vi "Auto备份.vi"() -> ()   [LabVIEW 2019]
uses:
  Global_Variable/A180648.vi
  Global_Variable/Global.vi
  Libraries/S7/S7.lvlib
  <userlib>/_MGI/1D Array/MGI Running Average/MGI Running Average(DBL).vi
  <userlib>/_MGI/1D Array/MGI Running Average/MGI Running Average(SGL).vi
  <userlib>/_MGI/1D Array/MGI Running Average/MGI Running Average(DBL[]).vi
panel:
  out "试验项_Event":refnum<user-event>
  out "NVH":bool=TRUE
  out "T1+T2":dbl
  out "T2":dbl
  out "T1":dbl
  out "吸收电流":sgl
  out "输出扭矩(大)":sgl
  out "输入扭矩":sgl
  out "力特性逆向去程":bool
  out "力特性正向去程":bool
  out "力特性逆向回程":bool
  out "力特性正向回程":bool
  out "逆向空载正向初始化":bool
  out "锁紧/开启初始化":bool
  out "功能正向初始化":bool
  out "功能逆向初始化":bool
  out "空载逆向初始化":bool
  out "空载正向初始化":bool
  out "布尔":bool=TRUE
  out "当前车速":i32
  out "试验项目":T1(tab)
  out "手柄锁紧力试验":cluster{dbl[], dbl[]}[](graph)
  out "手柄开启力试验":cluster{dbl[], dbl[]}[](graph)
  out "管柱推拉力试验":cluster{dbl[], dbl[]}[](graph)
  out "管柱保持力试验":cluster{dbl[], dbl[]}[](graph)
  out "锁紧/开启":cluster{dbl[], dbl[]}[](graph)
  out "逆向空载试验":cluster{dbl[], dbl[]}[](graph)
  out "振动2NHV-FFT":cluster{"f0":dbl, "df":dbl, "magnitude":dbl[]}[](graph)
  out "振动1NVH-FFT":cluster{"f0":dbl, "df":dbl, "magnitude":dbl[]}[](graph)
  in  "判定结果":bool[][](array[boolean])=[[TRUE]]
  in  "STEP":string
  # "车速1"
  # "车速2"
  # "车速3"
  # "车速4"
  # "车速5"
  # "车速6"
  # "车速1"
  # "车速2"
  # "车速3"
  # "车速4"
  # "车速5"
  # "车速6"
  # "."
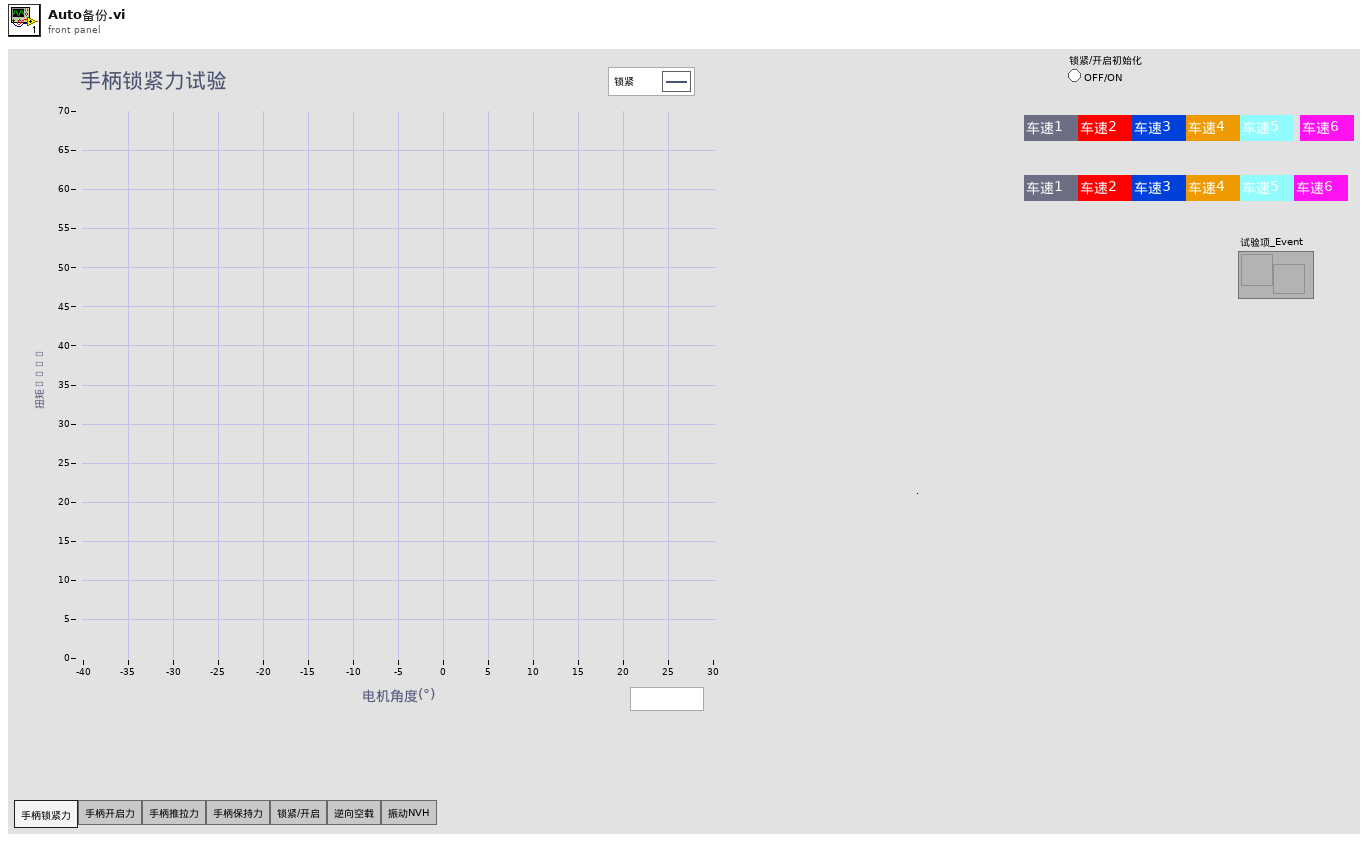
[diagram p1: front panel]
types:
  T1 = enum32{"手柄锁紧力", "手柄开启力", "手柄推拉力", "手柄保持力", "锁紧/开启", "逆向空载", "振动NVH"}
  T2 = enum32{"Invalid", "Standard", "Closed", "Hidden", "Minimized", "Maximized"}
  T3 = enum32{"手柄锁紧力", "手柄开启力", "手柄推拉力", "手柄保持力", "锁紧/开启", "逆向空载", "振动NVH", "完成"}
  T4 = cluster{"输入轴扭矩":dbl, "输出轴扭矩小量程":dbl, "输出轴扭矩大量程":dbl}
  T5 = cluster{"锁紧判断范围":cluster{"单位":string, "下限":dbl, "上限":dbl}}
  T6 = cluster{"开启判断范围":cluster{"单位":string, "下限":dbl, "上限":dbl}}
  T7 = cluster{"推拉力判断范围 ":cluster{"单位":string, "下限":dbl, "上限":dbl}}
  T8 = cluster{"保持力判断范围 ":cluster{"单位":string, "下限":dbl, "上限":dbl}, "保持力监控位移":cluster{"单位":string, "下限":dbl, "上限":dbl}}
  T9 = cluster{"输入旋转位移":sgl, "输入移载位移":sgl, "工装移载位移":sgl, "输入编码位移":sgl, "输入扭矩":sgl, "输出扭矩(小)":sgl, "输出扭矩(大)":sgl, "吸收电流":sgl}
  T10 = typedef "svc_Spectrum Info.ctl" = cluster{"channel name":string, "description":string, "x-axis units":T11, "spectral info":cluster{"spectrum type":T12, "linear/dB":enum16{"linear", "dB"}, "window":u16, "window size":i32, "FFT size":i32}, "engineering units":T13, "custom label":string, "dB reference [EU]":dbl, "peak units":enum16{"rms", "peak", "peak-peak"}, "weighting filter":T14, "spectral density?":bool, "unit label":string, "spectrum skewed?":bool, "complimentary spectrum units":T15}
  T11 = typedef "svc_X-Axis Units.ctl" = u16
  T12 = typedef "svc_Spectrum Type.ctl" = enum16{"FFT Spectrum [complex]", "Amplitude [Magnitude]", "Power [Magnitude^2]", "Cross Spectrum [complex]", "Frequency Response [Complex]"}
  T13 = typedef "svc_Engineering Units Text Ring.ctl" = u16
  T14 = typedef "svc_Weighting Filter Text Ring.ctl" = u16
  T15 = typedef "svc_Complimentary Spectrum Units.ctl" = enum16{"none", "radians", "degrees", "cycles", "imaginary"}
  T16 = cluster{"启用助力":dbl, "试验速度":dbl, "试验角度":dbl, "保护扭矩":dbl}
  T17 = typedef "lveventtype.ctl" = enum32{"Null", "Timeout", "Annotation Menu Selection", "Annotation Menu Selection?", "App Instance Close", "App Instance Close?", "Autoscale Range Change", "Bookmark Info Change", "Cell Edit", "Cell Edit?", "Cursor Grab", "Cursor Grab?", "Cursor Menu Selection", "Cursor Menu Selection?", "Cursor Move", "Cursor Release", "Data Change", "Direction Change", "Display State Change", "Drag Ended", "Drag Enter", "Drag Leave", "Drag Over", "Drag Source Update", "Drag Starting", "Drag Starting?", "Drop", "Exec State Change", "Key Down", "Key Down?", "Key Repeat", "Key Repeat?", "Key Up", "Listbox Double Click", "Menu Activation?", "Menu Selection (App)", "Menu Selection? (App)", "Menu Selection (User)", "Mouse Down", "Mouse Down?", "Mouse Enter", "Mouse Leave", "Mouse Move", "Mouse Up", "Mouse Wheel", "NI Security User Change (App)", "Pane Size", "Panel Close", "Panel Close?", "Panel Resize", "Plot Attribute Change", "Scale Range Change", "Shortcut Menu Activation?", "Shortcut Menu Selection (App)", "Shortcut Menu Selection? (App)", "Shortcut Menu Selection (User)", "Tree Double Click", "Tree Drag", "Tree Drag?", "Tree Drop", "Tree Drop?", "Tree Item Close", "Tree Item Close?", "Tree Item Open", "Tree Item Open?", "User Event", "Value Change"}
  T18 = typedef "LVPoint32TypeDef.ctl" = cluster{"Horizontal":i32, "Vertical":i32}
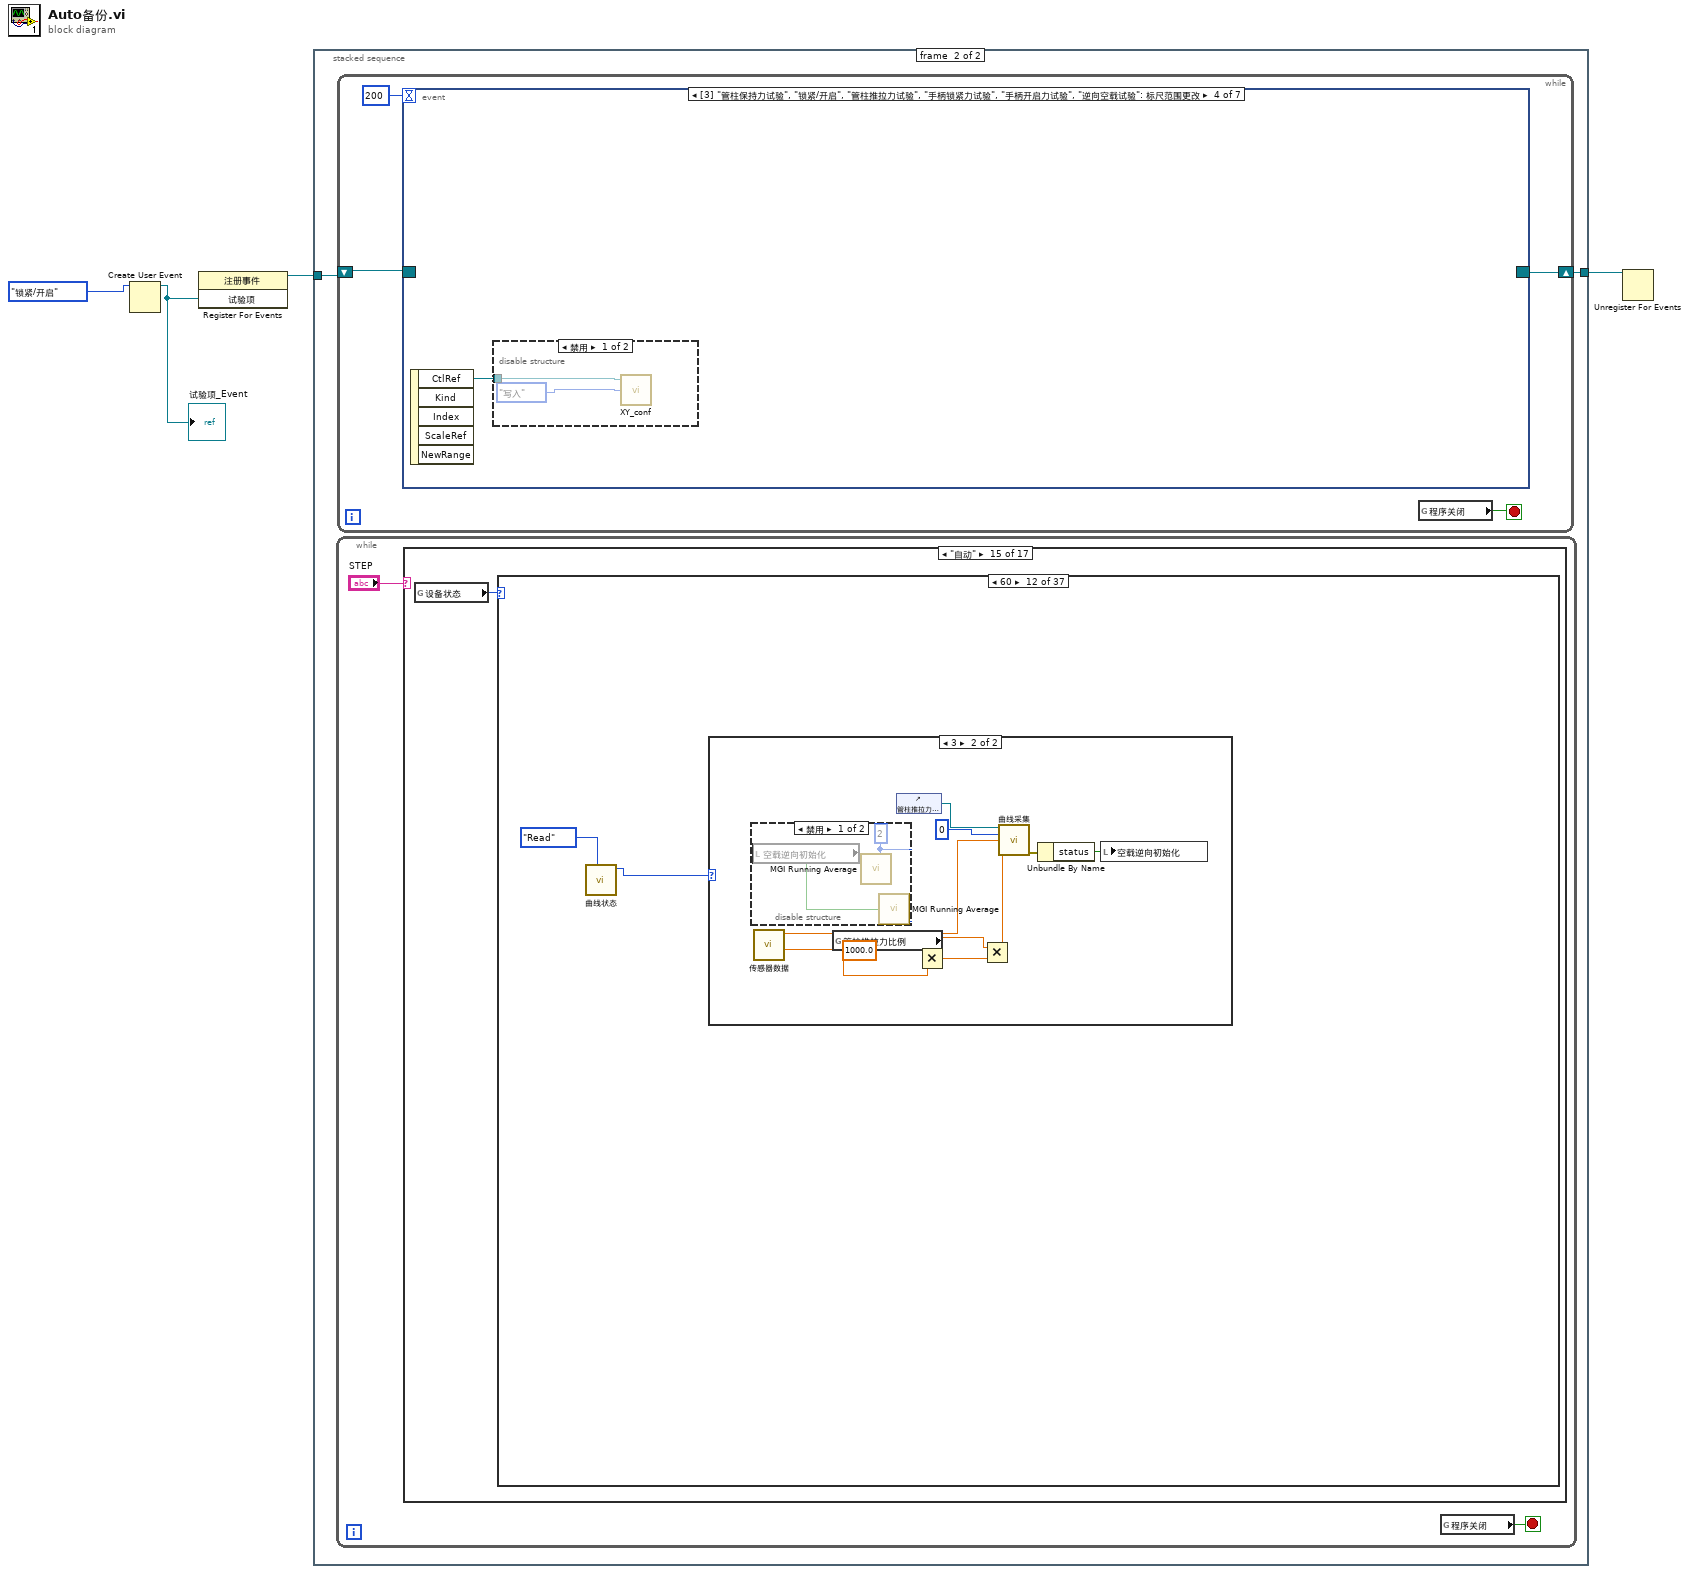
[diagram p0: block diagram]
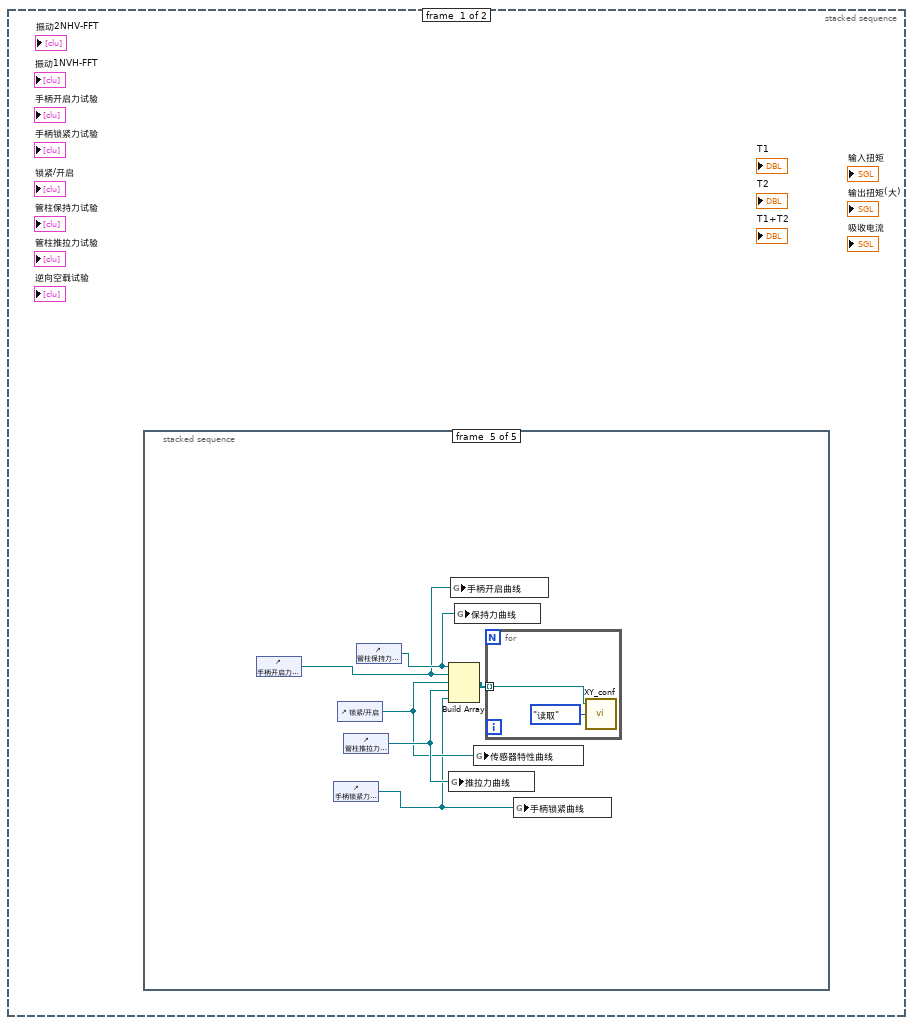
[diagram p2: hidden frame]
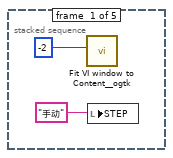
[diagram p3: hidden frame]
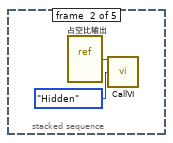
[diagram p4: hidden frame]
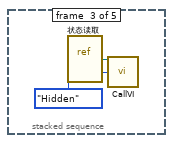
[diagram p5: hidden frame]
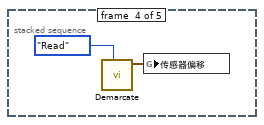
[diagram p6: hidden frame]
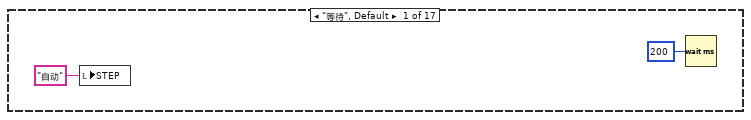
[diagram p7: hidden frame]
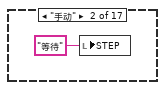
[diagram p8: hidden frame]
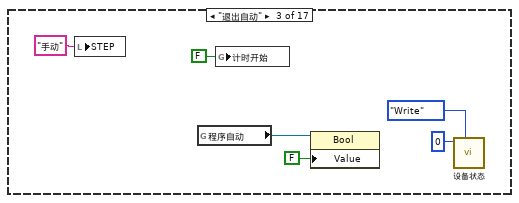
[diagram p9: hidden frame]
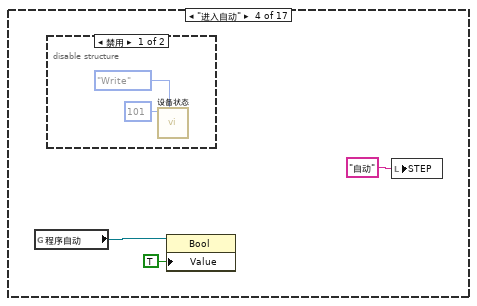
[diagram p10: hidden frame]
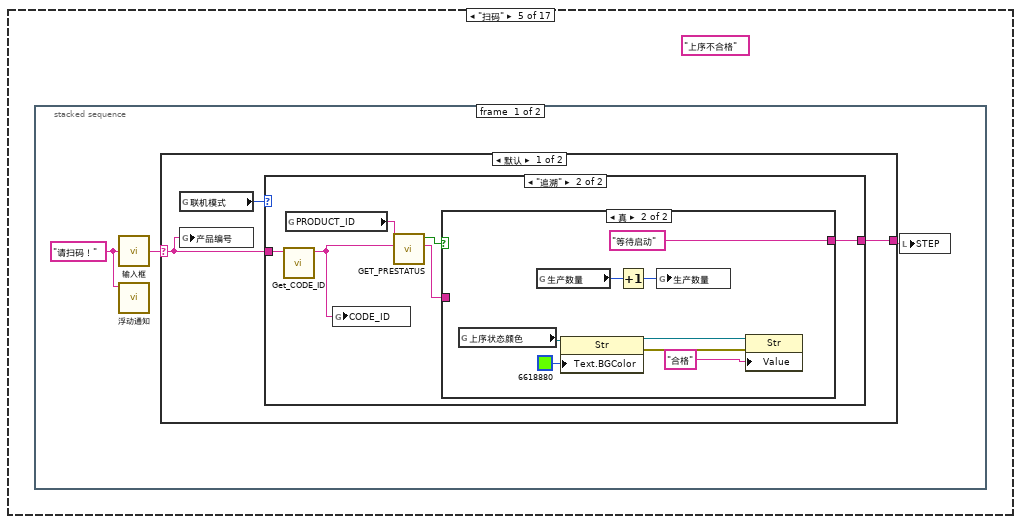
[diagram p12: hidden frame]
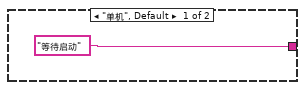
[diagram p13: hidden frame]
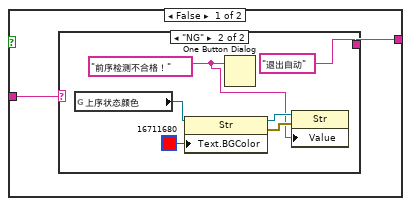
[diagram p14: hidden frame]
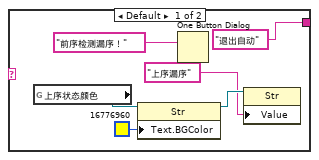
[diagram p15: hidden frame]
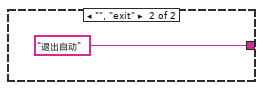
[diagram p16: hidden frame]
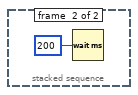
[diagram p17: hidden frame]
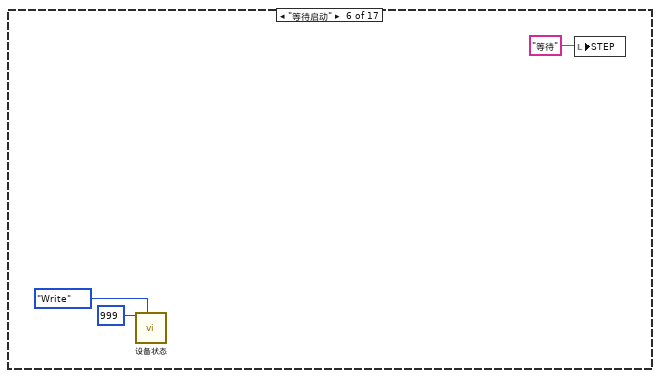
[diagram p18: hidden frame]
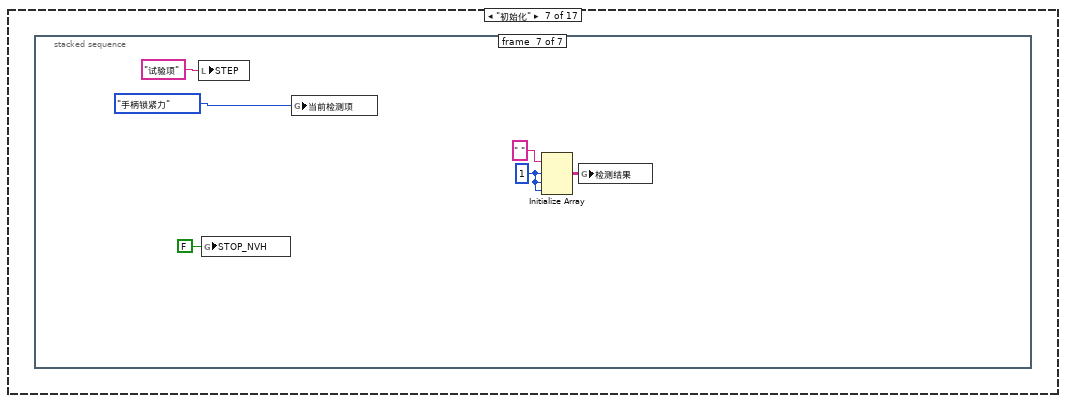
[diagram p19: hidden frame]
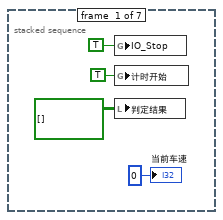
[diagram p20: hidden frame]
diagram:
  n1 = Create User Event(user event datatype=T1."锁紧/开启" ("试验项")) -> (user event=w1:refnum<user-event>)  [unwired: 1 in, 1 out]
  "试验项_Event" <- w1
  n2 = register-events(w1) -> (reference out=w2:refnum<event-registration>)  [unwired: 2 in, 1 out]
  n3 = stacked-sequence {
    tunnel: [_ w22] -> w4
    tunnel: w2 -> [_ w21]
    frame #0 {
      n4 = stacked-sequence {
        frame #0 {
          n5 = call <userlib>:"Fit VI window to Content__ogtk.vi"("border spacing (2 px)"=-2) -> ()  [unwired: 5 in, 2 out]
          n6 = local write "STEP"("手动" ("STEP")) -> ()
        }
        frame #1 {
          n7 = vi-ref "占空比输出.vi"() -> (w8:refnum<vi>)
          n8 = call "CallVI.vi"("VI引用"=w8, "状态"=T2."Hidden") -> ()  [unwired: 12 in, 2 out]
        }
        frame #2 {
          n9 = vi-ref "状态读取.vi"() -> (w10:refnum<vi>)
          n10 = call "CallVI.vi"("VI引用"=w10, "状态"=T2."Hidden") -> ()  [unwired: 12 in, 2 out]
        }
        frame #3 {
          n11 = call "Demarcate.vi"("Mode"=enum16{"Read", "Write"}."Read") -> ("Sensor OUT"=w12:T4)  [unwired: 9 in, 1 out]
          n12 = global write "传感器偏移.vi" "传感器偏移"(w12) -> ()
        }
        frame #4 {
          n13 = control-ref of="手柄开启力试验"() -> (w14:refnum<vi>)
          n14 = control-ref of="手柄锁紧力试验"() -> (w13:refnum<vi>)
          n15 = control-ref of="锁紧/开启"() -> (w15:refnum<vi>)
          n16 = control-ref of="管柱推拉力试验"() -> (w18:refnum<vi>)
          n17 = control-ref of="管柱保持力试验"() -> (w16:refnum<vi>)
          n18 = Build Array(w16, w14, w15, w18, w13) -> (w17:refnum<vi>[])
          n19 = global write "A180648.vi" "推拉力曲线"(w18) -> ()
          n20 = global write "A180648.vi" "手柄开启曲线"(w14) -> ()
          n21 = global write "A180648.vi" "保持力曲线"(w16) -> ()
          n22 = global write "A180648.vi" "传感器特性曲线"(w15) -> ()
          n23 = for {
            tunnel: w17 -> [w19] mode=indexing
            n24 = call "XY_conf.vi"("方式"=enum16{"写入", "读取"}."读取", "XY图引用"=w19) -> ()  [unwired: 3 in, 1 out]
          }
          n25 = global write "A180648.vi" "手柄锁紧曲线"(w13) -> ()
        }
      }
    }
    frame #1 {
      n26 = while {
        stop <- w24 stop-if-true
        n27 = case shown="\"自动\"" "STEP" {
          frame "等待", Default {
            n28 = local write "STEP"("自动" ("STEP")) -> ()
            n29 = Wait (ms)(milliseconds to wait=u32 200 ("等待时间（毫秒）")) -> ()  [unwired: 1 out]
          }
          frame "手动" {
            n30 = local write "STEP"("等待" ("STEP")) -> ()
          }
          frame "退出自动" {
            n31 = local write "STEP"("手动" ("STEP")) -> ()
            n32 = global read "Global.vi" "程序自动"() -> (w29:refnum<vi>)
            n33 = global write "Global.vi" "计时开始"(FALSE ("计时开始")) -> ()
            n34 = property class="Bool"(reference=w29, "Value"=FALSE) -> ()  [unwired: 1 in, 2 out]
            n35 = call "设备状态.vi"("枚举"=enum16{"Read", "Write"}."Write", "Status_Write"=i16 0) -> ()  [unwired: 9 in, 1 out]
          }
          frame "进入自动" {
            n36 = global read "Global.vi" "程序自动"() -> (w35:refnum<vi>)
            n37 = disable-structure shown="禁用" {
              frame Disabled {
                n38 = call "设备状态.vi"("枚举"=enum16{"Read", "Write"}."Write", "Status_Write"=i16 101) -> ()  [unwired: 9 in, 1 out]
              }
              frame Enabled {
              }
            }
            n39 = property class="Bool"(reference=w35, "Value"=TRUE) -> ()  [unwired: 1 in, 2 out]
            n40 = local write "STEP"("自动" ("STEP")) -> ()
          }
          frame "扫码" {
            (unwired) "上序不合格" ("上序状态")
            n41 = stacked-sequence {
              frame #0 {
                w40 = "请扫码！" ("提示信息")
                n42 = call "输入框.vi"("提示信息"=w40) -> ("条形码输出"=w41:string)
                n43 = call "浮动通知.vi"("通知内容"=w40) -> ()  [unwired: 11 in]
                n44 = case shown="默认" w41 {
                  selector: w41 -> [w43 _]
                  tunnel: [w44 "退出自动" ("State(s) in Front (\"\")")] -> w39
                  frame Default {
                    n45 = global read "Global.vi" "联机模式"() -> (w42:enum16{"单机", "追溯"})
                    n46 = global write "Global.vi" "产品编号"(w43) -> ()
                    n47 = case shown="\"追溯\"" w42 {
                      tunnel: ["等待启动" ("State(s) in Front (\"\")") w51] -> w44
                      tunnel: w43 -> [_ w48]
                      frame "单机", Default {
                      }
                      frame "追溯" {
                        n48 = call "Get_CODE_ID.vi"("CODE_MAIN"=w48) -> ("CODE_ID"=w47:string)  [unwired: 10 in]
                        n49 = global read "追溯Global.vi" "PRODUCT_ID"() -> (w50:string)
                        n50 = global write "追溯Global.vi" "CODE_ID"(w47) -> ()
                        n51 = call "GET_PRESTATUS.vi"("CODE_ID"=w47, "PRODUCT_ID"=w50) -> ("字符串"=w46:string, "OK?"=w49:bool)  [unwired: 8 in]
                        n52 = case shown="真" w49 {
                          tunnel: [w53 "等待启动" ("State(s) in Front (\"\")")] -> w51
                          tunnel: w46 -> [w52 _]
                          frame False {
                            n53 = case shown="\"NG\"" w52 {
                              tunnel: ["退出自动" ("State(s) in Front (\"\")") "退出自动" ("State(s) in Front (\"\")")] -> w53
                              frame Default {
                                n54 = global read "Global.vi" "上序状态颜色"() -> (w59:refnum<vi>)
                                n55 = property class="Str"(reference=w59, "Text.BGColor"=u32 16776960 ("文本.文本颜色:背景色")) -> (reference out=w55:refnum<vi>)  [unwired: 1 in, 1 out]
                                n56 = One Button Dialog(message="前序检测漏序！" ("消息")) -> ()  [unwired: 1 in, 1 out]
                                n57 = property class="Str"(reference=w55, "Value"="上序漏序" ("上序状态")) -> ()  [unwired: 1 in, 2 out]
                              }
                              frame "NG" {
                                w60 = "前序检测不合格！" ("消息")
                                n58 = global read "Global.vi" "上序状态颜色"() -> (w64:refnum<vi>)
                                n59 = property class="Str"(reference=w64, "Text.BGColor"=u32 16711680 ("文本.文本颜色:背景色")) -> (reference out=w62:refnum<vi>, error out=w61:errorcluster)  [unwired: 1 in]
                                n60 = One Button Dialog(message=w60) -> ()  [unwired: 1 in, 1 out]
                                n61 = property class="Str"(reference=w62, error in=w61, "Value"=w60) -> ()  [unwired: 2 out]
                              }
                            }
                          }
                          frame True {
                            n62 = global read "Global.vi" "上序状态颜色"() -> (w70:refnum<vi>)
                            n63 = global read "Global.vi" "生产数量"() -> (w71:i32)
                            n64 = property class="Str"(reference=w70, "Text.BGColor"=u32 6618880 ("文本.文本颜色:背景色")) -> (reference out=w68:refnum<vi>, error out=w67:errorcluster)  [unwired: 1 in]
                            n65 = Increment(x=w71) -> (x+1=w72:i32)
                            n66 = global write "Global.vi" "生产数量"(w72) -> ()
                            n67 = property class="Str"(reference=w68, error in=w67, "Value"="合格" ("上序状态")) -> ()  [unwired: 2 out]
                          }
                        }
                      }
                    }
                  }
                  frame "", "exit" {
                  }
                }
                n68 = local write "STEP"(w39) -> ()
              }
              frame #1 {
                n69 = Wait (ms)(milliseconds to wait=u32 200 ("等待时间（毫秒）")) -> ()  [unwired: 1 out]
              }
            }
          }
          frame "等待启动" {
            n70 = call "设备状态.vi"("枚举"=enum16{"Read", "Write"}."Write", "Status_Write"=i16 999 ("设备状态")) -> ()  [unwired: 9 in, 1 out]
            n71 = local write "STEP"("等待" ("STEP")) -> ()
          }
          frame "初始化" {
            n72 = stacked-sequence {
              frame #0 {
                n73 = global write "Global.vi" "IO_Stop"(TRUE ("IO_Stop")) -> ()
                n74 = global write "Global.vi" "计时开始"(TRUE ("计时开始")) -> ()
                n75 = local write "判定结果"(bool[][] [] ("判定结果")) -> ()
                "当前车速" <- 0 ("当前车速")
              }
              frame #1 {
                w86 = TRUE
                n76 = global read "Global.vi" "试验项目"() -> (w85:bool[])
                n77 = Index Array(array=w85, index=4 ("索引")) -> (element=w83:bool)
                n78 = case shown="假" w83 {
                  frame False {
                    n79 = local write "锁紧/开启初始化"(FALSE ("锁紧/开启初始化")) -> ()
                  }
                  frame True {
                    "锁紧/开启初始化" <- TRUE ("锁紧/开启初始化")
                  }
                }
                "逆向空载正向初始化" <- w86
                "空载正向初始化" <- w86
                "空载逆向初始化" <- w86
                "功能正向初始化" <- w86
                "功能逆向初始化" <- w86
                "力特性逆向去程" <- w86
                "力特性正向去程" <- w86
                "力特性逆向回程" <- w86
                "力特性正向回程" <- w86
              }
              frame #2 {
                n80 = for {
                  N: 24 -> [_]
                  tunnel: [cluster{dbl[], dbl[]} {[], []}] -> w90 mode=indexing
                  tunnel: [cluster{"f0":dbl, "df":dbl, "magnitude":dbl[]} {"f0"=0.0, "df"=0.0, "magnitude"=[]} ("power spectrum [dB EU]")] -> w89 mode=indexing
                }
                n81 = local write "管柱推拉力试验"(w90) -> ()
                n82 = local write "管柱保持力试验"(w90) -> ()
                n83 = local write "手柄锁紧力试验"(w90) -> ()
                n84 = local write "手柄开启力试验"(w90) -> ()
                n85 = local write "逆向空载试验"(w90) -> ()
                n86 = local write "锁紧/开启"(w90) -> ()
                n87 = local write "振动2NHV-FFT"(w89) -> ()
                n88 = local write "振动1NVH-FFT"(w89) -> ()
              }
              frame #3 {
                n89 = global read "Global.vi" "Result"() -> (w96:refnum<vi>)
                n90 = property class="Tbl"(reference=w96, "Value"=string[][] []) -> (reference out=w97:refnum<vi>, error out=w98:errorcluster)  [unwired: 1 in]
                n91 = property class="Tbl"(reference=w97, error in=w98, "Row Headers[]"=string[] [] ("列首字符串[]")) -> ()  [unwired: 2 out]
              }
              frame #4 {
                n92 = global read "A180648.vi" "LED-手柄锁紧力"() -> (w100:refnum<vi>)
                n93 = global read "A180648.vi" "LED-手柄开启力"() -> (w101:refnum<vi>)
                n94 = global read "A180648.vi" "LED-推拉力"() -> (w103:refnum<vi>)
                n95 = global read "A180648.vi" "LED-保持力"() -> (w99:refnum<vi>)
                n96 = Build Array(w100, w101, w103, w99) -> (w102:refnum<vi>[])
                n97 = for {
                  tunnel: w102 -> [w104] mode=indexing
                  n98 = property class="Bool"(reference=w104, "Colors [4]"=cluster{u32, u32}[] [{12369084, 12369084}] ("颜色[4]")) -> ()  [unwired: 1 in, 2 out]
                }
              }
              frame #5 {
                n99 = global read "Global.vi" "启用CAN"() -> (w106:bool)
                n100 = case shown="真" w106 {
                  frame False {
                  }
                  frame True {
                    n101 = call "循环发送CAN.vi"() -> ()  [unwired: 11 in, 1 out]
                  }
                }
              }
              frame #6 {
                w109 = 1 ("维数大小")
                n102 = local write "STEP"("试验项" ("STEP")) -> ()
                n103 = global write "Global.vi" "STOP_NVH"(FALSE ("STOP_NVH")) -> ()
                n104 = global write "A180648.vi" "当前检测项"(T3."手柄锁紧力" ("值(信号)")) -> ()
                n105 = Initialize Array(" " ("字符串"), w109, w109, w109) -> (w111:string[][][])
                n106 = global write "A180648.vi" "检测结果"(w111) -> ()
              }
            }
          }
          frame "试验项" {
            n107 = global read "A180648.vi" "当前检测项"() -> (w113:T3)
            n108 = case shown="\"完成\"" w113 {
              selector: w113 -> [w115 _]
              tunnel: [w118 "报表" ("STEP")] -> w114
              frame "手柄锁紧力", Default {
                n109 = global read "Global.vi" "试验项目"() -> (w116:bool[])
                n110 = Index Array(array=w116, index=w115) -> (element=w117:bool)
                n111 = case shown="真" w117 {
                  tunnel: ["试验项" ("字符串") w125] -> w118
                  tunnel: w115 -> [_ w126]
                  frame False {
                    n112 = global read "A180648.vi" "当前检测项"() -> (w123:T3)
                    n113 = Increment(x=w123) -> (x+1=w122:T3)
                    n114 = global write "A180648.vi" "当前检测项"(w122) -> ()
                    n115 = local read "判定结果"() -> (w119:bool[][])
                    n116 = Build Array (concatenate)(w119, bool[] [FALSE] ("判定结果")) -> (w120:bool[][])
                    n117 = local write "判定结果"(w120) -> ()
                  }
                  frame True {
                    n118 = case shown="\"手柄推拉力\"" w126 {
                      tunnel: ["手柄锁紧力" ("STEP") "手柄开启力" ("STEP") "手柄推拉力" ("STEP") "手柄保持力" ("STEP") "套输入轴花键" ("STEP") w153 "退输入轴花键" ("STEP")] -> w125
                      frame "手柄锁紧力", Default {
                        n119 = call "浮动通知.vi"("通知内容"="手柄锁紧力试验") -> ()  [unwired: 11 in]
                        n120 = property on="试验项目" class="TabCtl (严格)"("Val(Sgnl)"=T1."手柄锁紧力" ("值(信号)")) -> ()  [unwired: 2 in, 2 out]
                      }
                      frame "手柄开启力" {
                        n121 = call "浮动通知.vi"("通知内容"="手柄开启力试验") -> ()  [unwired: 11 in]
                        n122 = property on="试验项目" class="TabCtl (严格)"("Val(Sgnl)"=T1."手柄开启力" ("值(信号)")) -> ()  [unwired: 2 in, 2 out]
                      }
                      frame "手柄推拉力" {
                        n123 = call "浮动通知.vi"("通知内容"="管柱推拉力试验") -> ()  [unwired: 11 in]
                        n124 = property on="试验项目" class="TabCtl (严格)"("Val(Sgnl)"=T1."手柄推拉力" ("值(信号)")) -> ()  [unwired: 2 in, 2 out]
                      }
                      frame "手柄保持力" {
                        n125 = call "浮动通知.vi"("通知内容"="管柱保持力试验") -> ()  [unwired: 11 in]
                        n126 = property on="试验项目" class="TabCtl (严格)"("Val(Sgnl)"=T1."手柄保持力" ("值(信号)")) -> ()  [unwired: 2 in, 2 out]
                      }
                      frame "完成" {
                        n127 = for {
                          tunnel: sgl[] [1.0, 15.0] ("力特性参数") -> [w142] mode=indexing
                          i -> [w145]
                          w150 = u16 2 items=["byte", "word", "Dword"] ("数据类型")
                          w152 = u8 132 items=["I/O (P)"=128, "Input (I)"=129, "Output (Q)"=130, "Bit Memory (M)"=131, "Data (DB)"=132, "Instance Data (DI)"=133, "Local Data (L)"=134, "Predecessor Local Data (VL)"=135] ("寄存器类型")
                          n128 = Type Cast(type=u32 0 ("写入地址"), x=w142) -> (*(type *) &x=w148:u32)
                          n129 = Multiply(x=w145, y=4) -> (x*y=w146:i32)
                          n130 = Add(x=u32 152 ("写入地址"), y=w146) -> (x+y=w143:u32)
                          n131 = call "Write_Data.vi"("DB #"=u16 7, "寄存器类型"=w152, "写入数据"=w148, "数据类型"=w150, "写入地址"=w143) -> ()  [unwired: 4 in, 3 out]
                        }
                        n132 = call "浮动通知.vi"("通知内容"="传感器特性试验") -> ()  [unwired: 11 in]
                      }
                      frame "振动NVH" {
                        n133 = call "浮动通知.vi"("通知内容"="振动NVH试验") -> ()  [unwired: 11 in]
                        n134 = local read "NVH"() -> (w156:bool)
                        n135 = Select(t="判定" ("STEP"), s=w156, f="退输入轴花键" ("STEP")) -> (s? t:f=w153:string)
                      }
                      frame "逆向空载" {
                        n136 = call "浮动通知.vi"("通知内容"="逆向空载试验") -> ()  [unwired: 11 in]
                      }
                    }
                  }
                }
              }
              frame "完成" {
                n137 = call "浮动通知.vi"("通知内容"="试验完成") -> ()  [unwired: 11 in]
                n138 = call "设备状态.vi"("枚举"=enum16{"Read", "Write"}."Write", "Status_Write"=i16 100 ("设备状态")) -> ()  [unwired: 9 in, 1 out]
              }
            }
            n139 = local write "STEP"(w114) -> ()
          }
          frame "判定" {
            n140 = stacked-sequence {
              frame #0 {
                n141 = global read "A180648.vi" "当前检测项"() -> (w164:T3)
                n142 = case shown="\"手柄开启力\"" w164 {
                  frame "完成", Default {
                  }
                  frame "手柄锁紧力" {
                    n143 = global read "判定参数.vi" "锁紧判定参数"() -> (w176:T5)
                    n144 = local read "手柄锁紧力试验"() -> (w177:cluster{dbl[], dbl[]}[])
                    n145 = global read "A180648.vi" "LED-手柄锁紧力"() -> (w171:refnum<vi>)
                    n146 = global read "Global.vi" "Result"() -> (w175:refnum<vi>)
                    n147 = call "锁紧试验判定.vi"("Result"=w175, "判定参数"=w176, "XY曲线"=w177) -> ("判定项长度"=w166:i32, "OK？"=w165:bool)  [unwired: 7 in]
                    n148 = Select(t=cluster{u32, u32}[] [{6618880, 6618880}, {6618880, 6618880}, {6618880, 6618880}, {6618880, 6618880}] ("颜色[4]"), s=w165, f=cluster{u32, u32}[] [{16711680, 16711680}, {16711680, 16711680}, {16711680, 16711680}, {16711680, 16711680}] ("颜色[4]")) -> (s? t:f=w172:cluster{u32, u32}[])
                    n149 = property class="Bool"(reference=w171, "Colors [4]"=w172) -> ()  [unwired: 1 in, 2 out]
                    n150 = local read "判定结果"() -> (w167:bool[][])
                    n151 = Build Array(TRUE, w165) -> (w170:bool[])
                    n152 = global write "判定参数.vi" "锁紧判定长度"(w166) -> ()
                    n153 = Build Array (concatenate)(w167, w170) -> (w168:bool[][])
                    n154 = case shown="假" w165 {
                      frame False {
                        n155 = call "合格状态.vi"("枚举"=enum16{"Read", "Write"}."Write", "起始地址"=u32 180, "Status_Write"=i16 2) -> ()  [unwired: 8 in, 1 out]
                      }
                      frame True {
                        n156 = call "合格状态.vi"("枚举"=enum16{"Read", "Write"}."Write", "起始地址"=u32 180, "Status_Write"=i16 1) -> ()  [unwired: 8 in, 1 out]
                      }
                    }
                    n157 = local write "判定结果"(w168) -> ()
                  }
                  frame "手柄开启力" {
                    n158 = global read "A180648.vi" "LED-手柄开启力"() -> (w191:refnum<vi>)
                    n159 = global read "判定参数.vi" "开启判定参数"() -> (w196:T6)
                    n160 = local read "手柄开启力试验"() -> (w197:cluster{dbl[], dbl[]}[])
                    n161 = global read "Global.vi" "Result"() -> (w195:refnum<vi>)
                    n162 = call "开启试验判定.vi"("Result"=w195, "判定参数"=w196, "XY曲线"=w197) -> ("判定项长度"=w186:i32, "OK？"=w184:bool)  [unwired: 7 in]
                    n163 = Select(t=cluster{u32, u32}[] [{6618880, 6618880}, {6618880, 6618880}, {6618880, 6618880}, {6618880, 6618880}] ("颜色[4]"), s=w184, f=cluster{u32, u32}[] [{16711680, 16711680}, {16711680, 16711680}, {16711680, 16711680}, {16711680, 16711680}] ("颜色[4]")) -> (s? t:f=w192:cluster{u32, u32}[])
                    n164 = property class="Bool"(reference=w191, "Colors [4]"=w192) -> ()  [unwired: 1 in, 2 out]
                    n165 = local read "判定结果"() -> (w187:bool[][])
                    n166 = global write "判定参数.vi" "开启判定长度"(w186) -> ()
                    n167 = Build Array(TRUE, w184) -> (w190:bool[])
                    n168 = Build Array (concatenate)(w187, w190) -> (w188:bool[][])
                    n169 = case shown="假" w184 {
                      frame False {
                        n170 = call "合格状态.vi"("枚举"=enum16{"Read", "Write"}."Write", "起始地址"=u32 76, "Status_Write"=i16 2) -> ()  [unwired: 8 in, 1 out]
                      }
                      frame True {
                        n171 = call "合格状态.vi"("枚举"=enum16{"Read", "Write"}."Write", "起始地址"=u32 76, "Status_Write"=i16 1) -> ()  [unwired: 8 in, 1 out]
                      }
                    }
                    n172 = local write "判定结果"(w188) -> ()
                    "NVH" <- TRUE
                  }
                  frame "手柄推拉力" {
                    n173 = global read "判定参数.vi" "推拉力判定参数"() -> (w207:T7)
                    n174 = local read "管柱推拉力试验"() -> (w216:cluster{dbl[], dbl[]}[])
                    n175 = global read "A180648.vi" "LED-推拉力"() -> (w214:refnum<vi>)
                    n176 = global read "Global.vi" "Result"() -> (w205:refnum<vi>)
                    n177 = call "推拉力判定.vi"("Result"=w205, "判定参数"=w207, "XY曲线"=w216) -> ("判定项长度"=w206:i32, "OK？"=w204:bool)  [unwired: 7 in]
                    n178 = Select(t=cluster{u32, u32}[] [{6618880, 6618880}, {6618880, 6618880}, {6618880, 6618880}, {6618880, 6618880}] ("颜色[4]"), s=w204, f=cluster{u32, u32}[] [{16711680, 16711680}, {16711680, 16711680}, {16711680, 16711680}, {16711680, 16711680}] ("颜色[4]")) -> (s? t:f=w215:cluster{u32, u32}[])
                    n179 = property class="Bool"(reference=w214, "Colors [4]"=w215) -> ()  [unwired: 1 in, 2 out]
                    n180 = local read "判定结果"() -> (w208:bool[][])
                    n181 = global write "判定参数.vi" "推拉力判定长度"(w206) -> ()
                    n182 = case shown="真" w204 {
                      frame False {
                        n183 = call "合格状态.vi"("枚举"=enum16{"Read", "Write"}."Write", "起始地址"=u32 96, "Status_Write"=i16 2) -> ()  [unwired: 8 in, 1 out]
                      }
                      frame True {
                        n184 = call "合格状态.vi"("枚举"=enum16{"Read", "Write"}."Write", "起始地址"=u32 96, "Status_Write"=i16 1) -> ()  [unwired: 8 in, 1 out]
                      }
                    }
                    n185 = Build Array(TRUE, w204) -> (w211:bool[])
                    n186 = Build Array (concatenate)(w208, w211) -> (w209:bool[][])
                    n187 = local write "判定结果"(w209) -> ()
                  }
                  frame "手柄保持力" {
                    n188 = local read "管柱保持力试验"() -> (w237:cluster{dbl[], dbl[]}[])
                    n189 = global read "判定参数.vi" "保持力判定参数"() -> (w231:T8)
                    n190 = global read "判定参数.vi" "最小位移"() -> (w225:dbl)
                    n191 = global read "判定参数.vi" "最大位移"() -> (w224:dbl)
                    n192 = global read "A180648.vi" "LED-保持力"() -> (w235:refnum<vi>)
                    n193 = global read "Global.vi" "Result"() -> (w226:refnum<vi>)
                    n194 = call "保持力判定.vi"("Result"=w226, "最大位移"=w224, "最小位移"=w225, "判定参数"=w231, "XY曲线"=w237) -> ("判定项长度"=w227:i32, "OK？"=w223:bool)  [unwired: 5 in]
                    n195 = Select(t=cluster{u32, u32}[] [{6618880, 6618880}, {6618880, 6618880}, {6618880, 6618880}, {6618880, 6618880}] ("颜色[4]"), s=w223, f=cluster{u32, u32}[] [{16711680, 16711680}, {16711680, 16711680}, {16711680, 16711680}, {16711680, 16711680}] ("颜色[4]")) -> (s? t:f=w236:cluster{u32, u32}[])
                    n196 = property class="Bool"(reference=w235, "Colors [4]"=w236) -> ()  [unwired: 1 in, 2 out]
                    n197 = local read "判定结果"() -> (w232:bool[][])
                    n198 = case shown="真" w223 {
                      frame False {
                        n199 = call "合格状态.vi"("枚举"=enum16{"Read", "Write"}."Write", "起始地址"=u32 116, "Status_Write"=i16 2) -> ()  [unwired: 8 in, 1 out]
                      }
                      frame True {
                        n200 = call "合格状态.vi"("枚举"=enum16{"Read", "Write"}."Write", "起始地址"=u32 116, "Status_Write"=i16 1) -> ()  [unwired: 8 in, 1 out]
                      }
                    }
                    n201 = global write "判定参数.vi" "保持力判定长度"(w227) -> ()
                    n202 = Build Array(TRUE, w223) -> (w234:bool[])
                    n203 = Build Array (concatenate)(w232, w234) -> (w233:bool[][])
                    n204 = local write "判定结果"(w233) -> ()
                  }
                }
              }
              frame #1 {
                n205 = call "合格状态.vi"("枚举"=enum16{"Read", "Write"}."Read", "起始地址"=u32 76) -> ("Status_Read"=w244:i16)  [unwired: 9 in]
                n206 = case shown="1" w244 {
                  frame 2 {
                    n207 = call "合格状态.vi"("枚举"=enum16{"Read", "Write"}."Read", "起始地址"=u32 86) -> ("Status_Read"=w254:i16)  [unwired: 9 in]
                    n208 = call "合格状态.vi"("枚举"=enum16{"Read", "Write"}."Read", "起始地址"=u32 106) -> ("Status_Read"=w251:i16)  [unwired: 9 in]
                    n209 = call "合格状态.vi"("枚举"=enum16{"Read", "Write"}."Read", "起始地址"=u32 58) -> ("Status_Read"=w250:i16)  [unwired: 9 in]
                    n210 = Greater Or Equal?(x=w251, y=w250) -> (x >= y?=w248:bool)
                    n211 = Greater Or Equal?(x=w254, y=w250) -> (x >= y?=w249:bool)
                    n212 = Or(x=w249, y=w248) -> (x .or. y?=w247:bool)
                    n213 = case shown="假" w247 {
                      frame False {
                        n214 = local write "STEP"("等待" ("STEP")) -> ()
                        n215 = call "设备状态.vi"("枚举"=enum16{"Read", "Write"}."Write", "Status_Write"=i16 52) -> ()  [unwired: 9 in, 1 out]
                      }
                      frame True {
                        n216 = local write "STEP"("试验项" ("STEP")) -> ()
                        n217 = global write "A180648.vi" "当前检测项"(T3."完成" ("当前检测项")) -> ()
                      }
                    }
                  }
                  frame 1 {
                    n218 = call "合格状态.vi"("枚举"=enum16{"Read", "Write"}."Read", "起始地址"=u32 180) -> ("Status_Read"=w264:i16)  [unwired: 9 in]
                    n219 = case shown="1" w264 {
                      frame 0, Default {
                      }
                      frame 1 {
                        n220 = global read "A180648.vi" "当前检测项"() -> (w269:T3)
                        n221 = local write "STEP"("试验项" ("STEP")) -> ()
                        n222 = Increment(x=w269) -> (x+1=w268:T3)
                        n223 = global write "A180648.vi" "当前检测项"(w268) -> ()
                      }
                      frame 2 {
                        n224 = call "合格状态.vi"("枚举"=enum16{"Read", "Write"}."Read", "起始地址"=u32 86) -> ("Status_Read"=w281:i16)  [unwired: 9 in]
                        n225 = call "合格状态.vi"("枚举"=enum16{"Read", "Write"}."Read", "起始地址"=u32 106) -> ("Status_Read"=w280:i16)  [unwired: 9 in]
                        n226 = call "合格状态.vi"("枚举"=enum16{"Read", "Write"}."Read", "起始地址"=u32 58) -> ("Status_Read"=w279:i16)  [unwired: 9 in]
                        n227 = Greater Or Equal?(x=w280, y=w279) -> (x >= y?=w277:bool)
                        n228 = Greater Or Equal?(x=w281, y=w279) -> (x >= y?=w278:bool)
                        n229 = Or(x=w278, y=w277) -> (x .or. y?=w276:bool)
                        n230 = case shown="假" w276 {
                          frame False {
                            n231 = local write "STEP"("等待" ("STEP")) -> ()
                            n232 = call "设备状态.vi"("枚举"=enum16{"Read", "Write"}."Write", "Status_Write"=i16 52) -> ()  [unwired: 9 in, 1 out]
                          }
                          frame True {
                            n233 = local write "STEP"("试验项" ("STEP")) -> ()
                            n234 = global write "A180648.vi" "当前检测项"(T3."完成" ("当前检测项")) -> ()
                          }
                        }
                      }
                    }
                  }
                  frame 0, Default {
                    n235 = global read "A180648.vi" "当前检测项"() -> (w289:T3)
                    n236 = local write "STEP"("试验项" ("STEP")) -> ()
                    n237 = Increment(x=w289) -> (x+1=w288:T3)
                    n238 = global write "A180648.vi" "当前检测项"(w288) -> ()
                  }
                }
              }
            }
          }
          frame "手柄锁紧力" {
            n239 = disable-structure shown="禁用" {
              frame Disabled {
                n240 = call "设备状态.vi"() -> ("Status_Read"=w293:i16)  [unwired: 11 in]
                n241 = case shown="0, 默认" w293 {
                  frame 0, Default {
                  }
                  frame 103 {
                    n242 = global read "A180648.vi" "当前检测项"() -> (w295:T3)
                    n243 = case shown="\"手柄开启力\"" w295 {
                      tunnel: ["退输出轴花键" ("STEP") "套输出轴花键" ("STEP") "套输出轴花键" ("STEP") "套输出轴花键" ("STEP") "套输出轴花键" ("STEP")] -> w294
                      frame "手柄锁紧力", Default {
                      }
                      frame "手柄开启力" {
                      }
                      frame "手柄推拉力" {
                      }
                      frame "完成" {
                      }
                      frame "手柄保持力" {
                      }
                    }
                    n244 = local write "STEP"(w294) -> ()
                  }
                  frame 1024 {
                    n245 = local write "STEP"("退出自动" ("STEP")) -> ()
                  }
                }
              }
              frame Enabled {
              }
            }
            n246 = local write "STEP"("等待" ("STEP")) -> ()
            n247 = call "设备状态.vi"("枚举"=enum16{"Read", "Write"}."Write", "Status_Write"=i16 40 ("设备状态")) -> ()  [unwired: 9 in, 1 out]
          }
          frame "手柄开启力" {
            n248 = disable-structure shown="禁用" {
              frame Disabled {
                n249 = call "设备状态.vi"() -> ("Status_Read"=w305:i16)  [unwired: 11 in]
                n250 = case shown="105" w305 {
                  frame 0, Default {
                    n251 = call "设备状态.vi"("枚举"=enum16{"Read", "Write"}."Write", "Status_Write"=i16 104 ("设备状态")) -> ()  [unwired: 9 in, 1 out]
                  }
                  frame 105 {
                    n252 = global read "A180648.vi" "当前检测项"() -> (w309:T3)
                    n253 = case shown="\"完成\"" w309 {
                      tunnel: ["自动" ("STEP") "退输出轴花键" ("STEP") "套输出轴花键" ("STEP") "退输出轴花键" ("STEP")] -> w308
                      frame Default {
                      }
                      frame "振动NVH" {
                      }
                      frame "逆向空载" {
                      }
                      frame "完成" {
                      }
                    }
                    n254 = local write "STEP"(w308) -> ()
                  }
                  frame 1024 {
                    n255 = local write "STEP"("退出自动" ("STEP")) -> ()
                  }
                }
              }
              frame Enabled {
              }
            }
            n256 = local write "STEP"("等待" ("STEP")) -> ()
            n257 = call "设备状态.vi"("枚举"=enum16{"Read", "Write"}."Write", "Status_Write"=i16 50 ("设备状态")) -> ()  [unwired: 9 in, 1 out]
          }
          frame "手柄推拉力" {
            n258 = disable-structure shown="禁用" {
              frame Disabled {
                n259 = call "设备状态.vi"() -> ("Status_Read"=w318:i16)  [unwired: 11 in]
                n260 = case shown="107" w318 {
                  frame 0, Default {
                    n261 = call "设备状态.vi"("枚举"=enum16{"Read", "Write"}."Write", "Status_Write"=i16 106 ("设备状态")) -> ()  [unwired: 9 in, 1 out]
                  }
                  frame 107 {
                    n262 = local write "STEP"("设置输出轴模式" ("STEP")) -> ()
                  }
                  frame 1024 {
                    n263 = local write "STEP"("退出自动" ("STEP")) -> ()
                  }
                }
              }
              frame Enabled {
              }
            }
            n264 = local write "STEP"("等待" ("STEP")) -> ()
            n265 = call "设备状态.vi"("枚举"=enum16{"Read", "Write"}."Write", "Status_Write"=i16 60 ("设备状态")) -> ()  [unwired: 9 in, 1 out]
          }
          frame "手柄保持力" {
            n266 = disable-structure shown="禁用" {
              frame Disabled {
                n267 = call "设备状态.vi"() -> ("Status_Read"=w326:i16)  [unwired: 11 in]
                n268 = case shown="109" w326 {
                  frame 0, Default {
                    n269 = call "设备状态.vi"("枚举"=enum16{"Read", "Write"}."Write", "Status_Write"=i16 108 ("设备状态")) -> ()  [unwired: 9 in, 1 out]
                  }
                  frame 109 {
                    n270 = global read "A180648.vi" "当前检测项"() -> (w329:T3)
                    n271 = case shown="默认" w329 {
                      tunnel: ["自动" ("STEP") "自动" ("STEP") "报表" ("STEP") "自动" ("STEP")] -> w330
                      frame Default {
                      }
                      frame "振动NVH" {
                        n272 = call "设备状态.vi"("枚举"=enum16{"Read", "Write"}."Write", "Status_Write"=i16 142 ("设备状态")) -> ()  [unwired: 9 in, 1 out]
                      }
                      frame "完成" {
                        n273 = call "浮动通知.vi"("通知内容"="检测完成！" ("Status")) -> ()  [unwired: 11 in]
                        n274 = call "设备状态.vi"("枚举"=enum16{"Read", "Write"}."Write", "Status_Write"=i16 160) -> ()  [unwired: 9 in, 1 out]
                      }
                      frame "手柄锁紧力" {
                        n275 = call "设备状态.vi"("枚举"=enum16{"Read", "Write"}."Write", "Status_Write"=i16 112) -> ()  [unwired: 9 in, 1 out]
                      }
                    }
                    n276 = local write "STEP"(w330) -> ()
                  }
                  frame 110 {
                    n277 = local write "STEP"("退出自动" ("STEP")) -> ()
                  }
                }
              }
              frame Enabled {
              }
            }
            n278 = local write "STEP"("等待" ("STEP")) -> ()
            n279 = call "设备状态.vi"("枚举"=enum16{"Read", "Write"}."Write", "Status_Write"=i16 70 ("设备状态")) -> ()  [unwired: 9 in, 1 out]
          }
          frame "设置输出轴模式" {
            n280 = global read "A180648.vi" "当前检测项"() -> (w344:T3)
            n281 = case shown="\"手柄保持力\"" w344 {
              tunnel: ["自动" ("STEP") "自动" ("STEP") "自动" ("STEP") "自动" ("STEP") "自动" ("STEP") "自动" ("STEP")] -> w343
              frame Default {
              }
              frame "手柄开启力" {
                n282 = stacked-sequence {
                  frame #0 {
                    n283 = call "设备状态.vi"("枚举"=enum16{"Read", "Write"}."Write", "Status_Write"=i16 122 ("设备状态")) -> ()  [unwired: 9 in, 1 out]
                  }
                  frame #1 {
                    n284 = Wait (ms)(milliseconds to wait=u32 500 ("等待时间（毫秒）")) -> ()  [unwired: 1 out]
                  }
                  frame #2 {
                  }
                }
              }
              frame "手柄推拉力" {
                n285 = call "设备状态.vi"("枚举"=enum16{"Read", "Write"}."Write", "Status_Write"=i16 130 ("设备状态")) -> ()  [unwired: 9 in, 1 out]
              }
              frame "完成" {
                n286 = call "设备状态.vi"("枚举"=enum16{"Read", "Write"}."Write", "Status_Write"=i16 130 ("设备状态")) -> ()  [unwired: 9 in, 1 out]
              }
              frame "逆向空载" {
                n287 = call "设备状态.vi"("枚举"=enum16{"Read", "Write"}."Write", "Status_Write"=i16 152 ("设备状态")) -> ()  [unwired: 9 in, 1 out]
              }
              frame "手柄保持力" {
                n288 = call "设备状态.vi"("枚举"=enum16{"Read", "Write"}."Write", "Status_Write"=i16 130 ("设备状态")) -> ()  [unwired: 9 in, 1 out]
              }
            }
            n289 = local write "STEP"(w343) -> ()
          }
          frame "自动" {
            n290 = global read "Global.vi" "设备状态"() -> (w362:i16)
            n291 = case shown="60" w362 {
              frame -128 {
                n292 = global write "Global.vi" "计时开始"(FALSE ("计时开始")) -> ()
                n293 = call "浮动通知.vi"("通知内容"="复位中……" ("Status")) -> ()  [unwired: 11 in]
              }
              frame 0 {
                n294 = global write "Global.vi" "计时开始"(FALSE ("计时开始")) -> ()
                n295 = call "浮动通知.vi"("通知内容"="手动状态！" ("Status")) -> ()  [unwired: 11 in]
              }
              frame 1 {
                n296 = call "浮动通知.vi"("通知内容"="请复位！" ("Status")) -> ()  [unwired: 11 in]
              }
              frame 4 {
                n297 = call "浮动通知.vi"("通知内容"="复位完成" ("Status")) -> ()  [unwired: 11 in]
                n298 = global write "Global.vi" "计时开始"(FALSE ("计时开始")) -> ()
              }
              frame 8 {
                n299 = call "浮动通知.vi"("通知内容"="程序停止！" ("Status")) -> ()  [unwired: 11 in]
              }
              frame 40 {
                n300 = call "曲线状态.vi"("枚举"=enum16{"Read", "Write"}."Read") -> ("Status_Read"=w372:i16)  [unwired: 10 in]
                n301 = case shown="2" w372 {
                  frame 0, Default {
                  }
                  frame 2 {
                    n302 = call "传感器数据.vi"() -> ("电机角度"=w374:sgl, "扭矩"=w373:sgl)  [unwired: 6 in, 4 out]
                    n303 = local read "空载正向初始化"() -> (w380:bool)
                    n304 = local read "锁紧/开启初始化"() -> (w375:bool)
                    n305 = control-ref of="手柄锁紧力试验"() -> (w379:refnum<vi>)
                    n306 = call "曲线采集.vi"("曲线引用"=w379, "曲线索引"=0, "X"=w374, "Y"=w373) -> ("错误输出"=w377:errorcluster)  [unwired: 10 in, 1 out]
                    n307 = disable-structure shown="禁用" {
                      disable-tunnel: w380 -> [w386 _]
                      frame Disabled {
                        w385 = 2 ("Averaging Size")
                        n308 = call-poly <userlib>:"MGI Running Average.vi"("Averaging Size"=w385, "Initialize? (F)"=w386) -> ()  [unwired: 9 in, 1 out]
                        n309 = call-poly <userlib>:"MGI Running Average.vi"("Averaging Size"=w385, "Initialize? (F)"=w386) -> ()  [unwired: 9 in, 1 out]
                      }
                      frame Enabled {
                      }
                    }
                    n310 = Unbundle By Name(w377) -> ("status"=w376:bool)
                    n311 = local write "空载正向初始化"(w376) -> ()
                    n312 = case shown="真" w375 {
                      tunnel: w374 -> [_ w382]
                      tunnel: w373 -> [_ w381]
                      frame False {
                      }
                      frame True {
                        n313 = control-ref of="锁紧/开启"() -> (w383:refnum<vi>)
                        n314 = call "曲线采集.vi"("曲线引用"=w383, "曲线索引"=0, "X"=w382, "Y"=w381) -> ()  [unwired: 10 in, 2 out]
                      }
                    }
                  }
                }
              }
              frame 41 {
                n315 = local write "STEP"("判定" ("STEP")) -> ()
              }
              frame 50 {
                n316 = call "曲线状态.vi"("枚举"=enum16{"Read", "Write"}."Read") -> ("Status_Read"=w389:i16)  [unwired: 10 in]
                n317 = case shown="1" w389 {
                  frame 0, Default {
                  }
                  frame 1 {
                    n318 = global read "A180648.vi" "手柄开启扭矩比例"() -> (w390:dbl)
                    n319 = call "传感器数据.vi"() -> ("电机角度"=w394:sgl, "扭矩"=w393:sgl)  [unwired: 6 in, 4 out]
                    n320 = disable-structure shown="禁用" {
                      disable-tunnel: [w407 _] -> w399
                      disable-tunnel: [w406 _] -> _
                      frame Disabled {
                        w406 = 2 ("Averaging Size")
                        n321 = local read "功能逆向初始化"() -> (w407:bool)
                        n322 = call-poly <userlib>:"MGI Running Average.vi"("Averaging Size"=w406, "Initialize? (F)"=w407) -> ()  [unwired: 9 in, 1 out]
                        n323 = call-poly <userlib>:"MGI Running Average.vi"("Averaging Size"=w406, "Initialize? (F)"=w407) -> ()  [unwired: 9 in, 1 out]
                      }
                      frame Enabled {
                      }
                    }
                    n324 = Multiply(x=w393, y=w390) -> (x*y=w391:dbl)
                    n325 = control-ref of="手柄开启力试验"() -> (w397:refnum<vi>)
                    n326 = disable-structure shown="禁用" {
                      disable-tunnel: w399 -> [w405 _]
                      disable-tunnel: _ -> [w404 _]
                      frame Disabled {
                        n327 = call-poly <userlib>:"MGI Running Average.vi"("Averaging Size"=w404, "Initialize? (F)"=w405) -> ()  [unwired: 9 in, 1 out]
                      }
                      frame Enabled {
                      }
                    }
                    n328 = call "曲线采集.vi"("曲线引用"=w397, "曲线索引"=0, "X"=w394, "Y"=w391) -> ("错误输出"=w396:errorcluster)  [unwired: 10 in, 1 out]
                    n329 = Unbundle By Name(w396) -> ("status"=w395:bool)
                    n330 = local read "锁紧/开启初始化"() -> (w392:bool)
                    n331 = local write "功能逆向初始化"(w395) -> ()
                    n332 = case shown="真" w392 {
                      tunnel: w394 -> [_ w401]
                      tunnel: w391 -> [_ w400]
                      frame False {
                      }
                      frame True {
                        n333 = control-ref of="锁紧/开启"() -> (w403:refnum<vi>)
                        n334 = call "曲线采集.vi"("曲线引用"=w403, "曲线索引"=1, "X"=w401, "Y"=w400) -> ()  [unwired: 10 in, 2 out]
                      }
                    }
                  }
                }
              }
              frame 51 {
                n335 = global write "Global.vi" "STOP_NVH"(TRUE ("STOP_NVH")) -> ()
                n336 = local write "STEP"("判定" ("STEP")) -> ()
              }
              frame 52 {
                n337 = call "浮动通知.vi"("通知内容"="手柄力不合格请调整！") -> ()  [unwired: 11 in]
              }
              frame 54 {
                n338 = call "浮动通知.vi"("通知内容"="调整后请点击触摸屏按钮继续") -> ()  [unwired: 11 in]
              }
              frame 60 {
                n339 = call "曲线状态.vi"("枚举"=enum16{"Read", "Write"}."Read") -> ("Status_Read"=w413:i16)  [unwired: 10 in]
                n340 = case shown="3" w413 {
                  frame 0, Default {
                  }
                  frame 3 {
                    n341 = disable-structure shown="禁用" {
                      frame Disabled {
                        w424 = 2 ("Averaging Size")
                        n342 = local read "空载逆向初始化"() -> (w425:bool)
                        n343 = call-poly <userlib>:"MGI Running Average.vi"("Averaging Size"=w424, "Initialize? (F)"=w425) -> ()  [unwired: 9 in, 1 out]
                        n344 = call-poly <userlib>:"MGI Running Average.vi"("Averaging Size"=w424, "Initialize? (F)"=w425) -> ()  [unwired: 9 in, 1 out]
                      }
                      frame Enabled {
                      }
                    }
                    n345 = call "传感器数据.vi"() -> ("拉压力"=w418:sgl, "电缸位移"=w419:sgl)  [unwired: 6 in, 4 out]
                    n346 = global read "A180648.vi" "管柱推拉力比例"() -> (w414:dbl)
                    n347 = control-ref of="管柱推拉力试验"() -> (w423:refnum<vi>)
                    n348 = Multiply(x=sgl 1000.0, y=w418) -> (x*y=w417:sgl)
                    n349 = Multiply(x=w414, y=w417) -> (x*y=w415:dbl)
                    n350 = call "曲线采集.vi"("曲线引用"=w423, "曲线索引"=0, "X"=w419, "Y"=w415) -> ("错误输出"=w421:errorcluster)  [unwired: 10 in, 1 out]
                    n351 = Unbundle By Name(w421) -> ("status"=w420:bool)
                    n352 = local write "空载逆向初始化"(w420) -> ()
                  }
                }
              }
              frame 61 {
                n353 = local write "STEP"("判定" ("STEP")) -> ()
              }
              frame 70 {
                n354 = call "曲线状态.vi"() -> ("Status_Read"=w427:i16)  [unwired: 11 in]
                n355 = disable-structure shown="禁用" {
                  disable-tunnel: _ -> [w434 _]
                  frame Disabled {
                    n356 = local read "当前车速"() -> (w436:i32)
                    n357 = global read "Global.vi" "传感器读数"() -> (w435:T9)
                    n358 = control-ref of="管柱推拉力试验"() -> (w437:refnum<vi>)
                    n359 = control-ref of="锁紧/开启"() -> (w438:refnum<vi>)
                    n360 = local read "力特性正向回程"() -> (w439:bool)
                    n361 = case shown="100" w436 {
                      selector: w436 -> [w461 _]
                      tunnel: w435 -> [w466 w482]
                      tunnel: w437 -> [w465 _]
                      tunnel: w438 -> [_ w480]
                      tunnel: w434 -> [w463 _]
                      tunnel: w439 -> [w452 w468]
                      tunnel: [FALSE FALSE] -> w440
                      tunnel: [w453 w472] -> w441
                      tunnel: [w455 _] -> w442
                      tunnel: [w454 _] -> w443
                      tunnel: [_ w471] -> w444
                      tunnel: [_ w470] -> w445
                      tunnel: [_ w469] -> w446
                      tunnel: 10 -> [w451 w467]
                      frame 0, Default {
                        n362 = Unbundle By Name(w466) -> ("输入扭矩"=w464:sgl, "输出扭矩(大)"=w450:sgl, "吸收电流"=w462:sgl)
                        n363 = Multiply(x=w461, y=4) -> (x*y=w458:i32)
                        n364 = Subtract(x=w450, y=sgl 0.0) -> (x-y=w448:sgl)
                        n365 = call-poly <userlib>:"MGI Running Average.vi"("Averaging Size"=w451, "Initialize? (F)"=w452, "Value"=w462) -> ("Average"=w454:sgl)  [unwired: 8 in]
                        n366 = call-poly <userlib>:"MGI Running Average.vi"("Averaging Size"=w451, "Initialize? (F)"=w452, "Value"=w464) -> ("Average"=w453:sgl)  [unwired: 8 in]
                        n367 = call-poly <userlib>:"MGI Running Average.vi"("Averaging Size"=w451, "Initialize? (F)"=w452, "Value"=w448) -> ("Average"=w455:sgl)  [unwired: 8 in]
                        n368 = Add(x=w458, y=1) -> (x+y=w457:i32)
                        n369 = call "曲线采集.vi"("曲线引用"=w463, "曲线索引"=w457, "X"=w453, "Y"=w454) -> ()  [unwired: 10 in, 2 out]
                        n370 = call "曲线采集.vi"("曲线引用"=w465, "曲线索引"=w457, "X"=w453, "Y"=w455) -> ()  [unwired: 10 in, 2 out]
                      }
                      frame 100 {
                        n371 = Unbundle By Name(w482) -> ("输入扭矩"=w481:sgl)
                        n372 = call "占空比.vi"() -> ("T1+T2"=w477:dbl, "T2"=w478:dbl, "T1"=w479:dbl)  [unwired: 9 in]
                        n373 = call-poly <userlib>:"MGI Running Average.vi"("Averaging Size"=w467, "Initialize? (F)"=w468, "Value"=w481) -> ("Average"=w472:sgl)  [unwired: 8 in]
                        n374 = call-poly <userlib>:"MGI Running Average.vi"("Averaging Size"=w467, "Initialize? (F)"=w468, "Value"=w477) -> ("Average"=w471:dbl)  [unwired: 8 in]
                        n375 = call-poly <userlib>:"MGI Running Average.vi"("Averaging Size"=w467, "Initialize? (F)"=w468, "Value"=w479) -> ("Average"=w469:dbl)  [unwired: 8 in]
                        n376 = call-poly <userlib>:"MGI Running Average.vi"("Averaging Size"=w467, "Initialize? (F)"=w468, "Value"=w478) -> ("Average"=w470:dbl)  [unwired: 8 in]
                        n377 = call "曲线采集.vi"("曲线引用"=w480, "曲线索引"=5, "X"=w472, "Y"=w471) -> ()  [unwired: 10 in, 2 out]
                        n378 = call "曲线采集.vi"("曲线引用"=w480, "曲线索引"=3, "X"=w472, "Y"=w469) -> ()  [unwired: 10 in, 2 out]
                        n379 = call "曲线采集.vi"("曲线引用"=w480, "曲线索引"=4, "X"=w472, "Y"=w470) -> ()  [unwired: 10 in, 2 out]
                      }
                    }
                    n380 = local write "力特性正向回程"(w440) -> ()
                    n381 = local write "吸收电流"(w443) -> ()
                    n382 = local write "输入扭矩"(w441) -> ()
                    n383 = local write "输出扭矩(大)"(w442) -> ()
                    n384 = local write "T1+T2"(w444) -> ()
                    n385 = local write "T1"(w446) -> ()
                    n386 = local write "T2"(w445) -> ()
                  }
                  frame Enabled {
                  }
                }
                n387 = case shown="4" w427 {
                  frame 0, Default {
                  }
                  frame 4 {
                    n388 = control-ref of="管柱保持力试验"() -> (w433:refnum<vi>)
                    n389 = call "传感器数据.vi"() -> ("拉压力"=w428:sgl, "电缸位移"=w431:sgl)  [unwired: 6 in, 4 out]
                    n390 = Multiply(x=sgl 1000.0, y=w428) -> (x*y=w430:sgl)
                    n391 = call "曲线采集.vi"("曲线引用"=w433, "曲线索引"=0, "X"=w431, "Y"=w430) -> ()  [unwired: 10 in, 2 out]
                  }
                }
              }
              frame 71 {
                n392 = local write "STEP"("判定" ("STEP")) -> ()
              }
              frame 100 {
                n393 = call "浮动通知.vi"("通知内容"="请放入产品后按启动夹紧产品！" ("Status")) -> ()  [unwired: 11 in]
              }
              frame 101 {
                n394 = local write "STEP"("扫码" ("STEP")) -> ()
              }
              frame 113 {
                n395 = call "设备状态.vi"("枚举"=enum16{"Read", "Write"}."Write", "Status_Write"=i16 114 ("设备状态")) -> ()  [unwired: 9 in, 1 out]
                n396 = local write "STEP"("等待" ("STEP")) -> ()
              }
              frame 122 {
                n397 = disable-structure shown="禁用" {
                  frame Disabled {
                    w490 = 2 ("Averaging Size")
                    n398 = local read "功能正向初始化"() -> (w489:bool)
                    n399 = call "传感器数据.vi"() -> ()  [unwired: 6 in, 6 out]
                    n400 = Unbundle By Name() -> ()  [unwired: 1 in, 3 out]
                    n401 = case shown="真" w489 {
                      frame False {
                      }
                      frame True {
                        n402 = vi-ref "NVH_TEST.vi"() -> (w498:refnum<vi>)
                        n403 = property class="VI"(reference=w498) -> (error out=w500:errorcluster, "Name"=w501:string)  [unwired: 1 in, 1 out]
                        n404 = control-ref of="振动2NHV-FFT"() -> (w494:refnum<vi>)
                        n405 = control-ref of="振动1NVH-FFT"() -> (w496:refnum<vi>)
                        n406 = Open VI Reference(type specifier VI Refnum (for type only)=refnum<vi> refnum, vi path=w501, options=128 ("调用并忽略输出"), error in (no error)=w500) -> (vi reference=w497:refnum<vi>)  [unwired: 2 in, 1 out]
                        n407 = call-by-ref "开始异步调用"(reference=w497, "振动NHV-FFT"=w494, "振动NVH-Order"=w496) -> (reference out=w504:refnum<vi>, error out=w502:errorcluster)  [unwired: 11 in]
                        n408 = Close Reference(reference=w504, error in (no error)=w502) -> (error out=w503:errorcluster)
                        n409 = call <vilib>:"Simple Error Handler.vi"("error in (no error)"=w503) -> ()  [unwired: 4 in, 5 out]
                      }
                    }
                    n410 = call-poly <userlib>:"MGI Running Average.vi"("Averaging Size"=w490, "Initialize? (F)"=w489) -> ("Average[i]"=w493:dbl[])  [unwired: 9 in]
                    n411 = call-poly <userlib>:"MGI Running Average.vi"("Averaging Size"=w490, "Initialize? (F)"=w489) -> ("Average[i]"=w492:dbl[])  [unwired: 9 in]
                    n412 = call-poly <userlib>:"MGI Running Average.vi"("Averaging Size"=w490, "Initialize? (F)"=w489) -> ("Average[i]"=w491:dbl[])  [unwired: 9 in]
                    n413 = Greater Or Equal To 0?(x=w493) -> ()  [unwired: 1 out]
                    n414 = case shown="真" {
                      selector: _ -> [_ _]
                      tunnel: w492 -> [_ _]
                      tunnel: w491 -> [_ _]
                      tunnel: w493 -> [_ _]
                      frame False {
                      }
                      frame True {
                        n415 = control-ref of="手柄开启力试验"() -> (w508:refnum<vi>)
                        n416 = call "曲线采集.vi"("曲线引用"=w508, "曲线索引"=0) -> ("错误输出"=w506:errorcluster)  [unwired: 12 in, 1 out]
                        n417 = call "曲线采集.vi"("曲线引用"=w508, "曲线索引"=2) -> ()  [unwired: 12 in, 2 out]
                        n418 = Unbundle By Name(w506) -> ("status"=w505:bool)
                        n419 = local write "功能正向初始化"(w505) -> ()
                      }
                    }
                  }
                  frame Enabled {
                  }
                }
              }
              frame 123 {
                n420 = stacked-sequence {
                  frame #0 {
                    n421 = call "设备状态.vi"("枚举"=enum16{"Read", "Write"}."Write", "Status_Write"=i16 124 ("设备状态")) -> ()  [unwired: 9 in, 1 out]
                  }
                  frame #1 {
                  }
                }
              }
              frame 130 {
                w512 = TRUE
                n422 = global read "A180648.vi" "当前检测项"() -> (w514:T3)
                n423 = case shown="\"完成\"" w514 {
                  tunnel: [0 100] -> w513
                  frame Default {
                    w517 = u16 2 items=["byte", "word", "Dword"] ("数据类型")
                    w518 = u8 132 items=["I/O (P)"=128, "Input (I)"=129, "Output (Q)"=130, "Bit Memory (M)"=131, "Data (DB)"=132, "Instance Data (DI)"=133, "Local Data (L)"=134, "Predecessor Local Data (VL)"=135] ("寄存器类型")
                    n424 = global read "A180648.vi" "车速"() -> (w524:sgl[])
                    n425 = Index Array(array=w524) -> (element=w523:sgl)  [unwired: 1 in]
                    n426 = Round Toward +Infinity(x=w523) -> (ceil(x): smallest int >= x=w522:sgl)
                    n427 = disable-structure shown="禁用" {
                      frame Disabled {
                        n428 = call-poly "模式选择.vi"("Max Torque"=200.0, "Velocity"=sgl 1.0) -> ()  [unwired: 9 in, 1 out]
                      }
                      frame Enabled {
                      }
                    }
                    n429 = Type Cast(type=u32 0, x=w523) -> (*(type *) &x=w525:u32)
                    n430 = To Unsigned Word Integer(number=w522) -> (unsigned 16bit integer=w521:u16)
                    n431 = call "Write_Data.vi"("DB #"=u16 7, "寄存器类型"=w518, "写入数据"=w525, "数据类型"=w517, "写入地址"=u32 160) -> ()  [unwired: 4 in, 3 out]
                    n432 = global write "A180648.vi" "当前车速"(w521) -> ()
                  }
                  frame "完成" {
                    w528 = u32 0
                    w530 = u16 2 items=["byte", "word", "Dword"] ("数据类型")
                    w533 = u8 132 items=["I/O (P)"=128, "Input (I)"=129, "Output (Q)"=130, "Bit Memory (M)"=131, "Data (DB)"=132, "Instance Data (DI)"=133, "Local Data (L)"=134, "Predecessor Local Data (VL)"=135] ("寄存器类型")
                    n433 = global write "A180648.vi" "当前车速"(w528) -> ()
                    n434 = call "Write_Data.vi"("DB #"=u16 7, "寄存器类型"=w533, "写入数据"=w528, "数据类型"=w530, "写入地址"=u32 160) -> ()  [unwired: 4 in, 3 out]
                  }
                }
                n435 = local write "力特性逆向回程"(w512) -> ()
                n436 = local write "力特性正向去程"(w512) -> ()
                n437 = local write "力特性逆向去程"(w512) -> ()
                n438 = local write "力特性正向回程"(w512) -> ()
                n439 = local write "当前车速"(w513) -> ()
              }
              frame 132 {
                n440 = disable-structure shown="禁用" {
                  frame Disabled {
                    n441 = control-ref of="管柱保持力试验"() -> (w539:refnum<vi>)
                    n442 = local read "当前车速"() -> (w536:i32)
                    n443 = global read "Global.vi" "传感器读数"() -> (w535:T9)
                    n444 = control-ref of="管柱推拉力试验"() -> (w537:refnum<vi>)
                    n445 = control-ref of="锁紧/开启"() -> (w538:refnum<vi>)
                    n446 = local read "力特性正向去程"() -> (w540:bool)
                    n447 = case shown="100" w536 {
                      selector: w536 -> [w558 _]
                      tunnel: w535 -> [w563 w573]
                      tunnel: w537 -> [w562 _]
                      tunnel: w538 -> [_ w571]
                      tunnel: w539 -> [w560 _]
                      tunnel: w540 -> [w549 w565]
                      tunnel: [FALSE FALSE] -> w541
                      tunnel: [w550 w566] -> w542
                      tunnel: [w552 _] -> _
                      tunnel: [w551 _] -> w543
                      tunnel: 10 -> [w548 w564]
                      frame 0, Default {
                        n448 = Unbundle By Name(w563) -> ("输入扭矩"=w561:sgl, "输出扭矩(大)"=w547:sgl, "吸收电流"=w559:sgl)
                        n449 = Multiply(x=w558, y=4) -> (x*y=w555:i32)
                        n450 = Subtract(x=w547, y=sgl 0.0) -> (x-y=w545:sgl)
                        n451 = call-poly <userlib>:"MGI Running Average.vi"("Averaging Size"=w548, "Initialize? (F)"=w549, "Value"=w559) -> ("Average"=w551:sgl)  [unwired: 8 in]
                        n452 = call-poly <userlib>:"MGI Running Average.vi"("Averaging Size"=w548, "Initialize? (F)"=w549, "Value"=w561) -> ("Average"=w550:sgl)  [unwired: 8 in]
                        n453 = call-poly <userlib>:"MGI Running Average.vi"("Averaging Size"=w548, "Initialize? (F)"=w549, "Value"=w545) -> ("Average"=w552:sgl)  [unwired: 8 in]
                        n454 = Add(x=w555, y=0) -> (x+y=w554:i32)
                        n455 = call "曲线采集.vi"("曲线引用"=w560, "曲线索引"=w554, "X"=w550, "Y"=w551) -> ()  [unwired: 10 in, 2 out]
                        n456 = call "曲线采集.vi"("曲线引用"=w562, "曲线索引"=w554, "X"=w550, "Y"=w552) -> ()  [unwired: 10 in, 2 out]
                      }
                      frame 100 {
                        n457 = Unbundle By Name(w573) -> ("输入扭矩"=w572:sgl)
                        n458 = call-poly <userlib>:"MGI Running Average.vi"("Averaging Size"=w564, "Initialize? (F)"=w565, "Value"=w572) -> ("Average"=w566:sgl)  [unwired: 8 in]
                        n459 = call-poly <userlib>:"MGI Running Average.vi"("Averaging Size"=w564, "Initialize? (F)"=w565) -> ()  [unwired: 9 in, 1 out]
                        n460 = call-poly <userlib>:"MGI Running Average.vi"("Averaging Size"=w564, "Initialize? (F)"=w565) -> ()  [unwired: 9 in, 1 out]
                        n461 = call-poly <userlib>:"MGI Running Average.vi"("Averaging Size"=w564, "Initialize? (F)"=w565) -> ()  [unwired: 9 in, 1 out]
                        n462 = call "曲线采集.vi"("曲线引用"=w571, "曲线索引"=2, "X"=w566) -> ()  [unwired: 11 in, 2 out]
                        n463 = call "曲线采集.vi"("曲线引用"=w571, "曲线索引"=0, "X"=w566) -> ()  [unwired: 11 in, 2 out]
                        n464 = call "曲线采集.vi"("曲线引用"=w571, "曲线索引"=1, "X"=w566) -> ()  [unwired: 11 in, 2 out]
                      }
                    }
                    n465 = local write "力特性正向去程"(w541) -> ()
                    n466 = local write "吸收电流"(w543) -> ()
                    n467 = local write "输入扭矩"(w542) -> ()
                  }
                  frame Enabled {
                  }
                }
                "布尔" <- TRUE ("布尔")
              }
              frame 133 {
                n468 = local write "STEP"("等待" ("STEP")) -> ()
                n469 = call "设备状态.vi"("枚举"=enum16{"Read", "Write"}."Write", "Status_Write"=i16 134 ("设备状态")) -> ()  [unwired: 9 in, 1 out]
                n470 = disable-structure shown="禁用" {
                  frame Disabled {
                    n471 = global read "A180648.vi" "当前检测项"() -> (w577:T3)
                    n472 = case shown="\"手柄推拉力\"" w577 {
                      frame Default {
                      }
                      frame "手柄推拉力" {
                        n473 = call-poly "模式选择.vi"("Max Torque"=200.0, "Velocity"=sgl -1.0) -> ()  [unwired: 9 in, 1 out]
                      }
                    }
                  }
                  frame Enabled {
                  }
                }
              }
              frame 136 {
                n474 = disable-structure shown="禁用" {
                  frame Disabled {
                    n475 = local read "力特性逆向去程"() -> (w585:bool)
                    n476 = control-ref of="管柱保持力试验"() -> (w584:refnum<vi>)
                    n477 = local read "当前车速"() -> (w581:i32)
                    n478 = global read "Global.vi" "传感器读数"() -> (w580:T9)
                    n479 = control-ref of="管柱推拉力试验"() -> (w582:refnum<vi>)
                    n480 = control-ref of="锁紧/开启"() -> (w583:refnum<vi>)
                    n481 = case shown="0, 默认" w581 {
                      selector: w581 -> [w607 _]
                      tunnel: w580 -> [w612 w628]
                      tunnel: w582 -> [w611 _]
                      tunnel: w583 -> [_ w626]
                      tunnel: w584 -> [w609 _]
                      tunnel: w585 -> [w598 w614]
                      tunnel: [FALSE FALSE] -> w586
                      tunnel: [w599 w618] -> w587
                      tunnel: [w601 _] -> w588
                      tunnel: [w600 _] -> w589
                      tunnel: [_ w617] -> w590
                      tunnel: [_ w616] -> w591
                      tunnel: [_ w615] -> w592
                      tunnel: 10 -> [w597 w613]
                      frame 0, Default {
                        n482 = Unbundle By Name(w612) -> ("输入扭矩"=w610:sgl, "输出扭矩(大)"=w596:sgl, "吸收电流"=w608:sgl)
                        n483 = Multiply(x=w607, y=4) -> (x*y=w604:i32)
                        n484 = Subtract(x=w596, y=sgl 0.0) -> (x-y=w595:sgl)
                        n485 = call-poly <userlib>:"MGI Running Average.vi"("Averaging Size"=w597, "Initialize? (F)"=w598, "Value"=w608) -> ("Average"=w600:sgl)  [unwired: 8 in]
                        n486 = call-poly <userlib>:"MGI Running Average.vi"("Averaging Size"=w597, "Initialize? (F)"=w598, "Value"=w610) -> ("Average"=w599:sgl)  [unwired: 8 in]
                        n487 = call-poly <userlib>:"MGI Running Average.vi"("Averaging Size"=w597, "Initialize? (F)"=w598, "Value"=w595) -> ("Average"=w601:sgl)  [unwired: 8 in]
                        n488 = Add(x=w604, y=2) -> (x+y=w603:i32)
                        n489 = call "曲线采集.vi"("曲线引用"=w609, "曲线索引"=w603, "X"=w599, "Y"=w600) -> ()  [unwired: 10 in, 2 out]
                        n490 = call "曲线采集.vi"("曲线引用"=w611, "曲线索引"=w603, "X"=w599, "Y"=w601) -> ()  [unwired: 10 in, 2 out]
                      }
                      frame 100 {
                        n491 = Unbundle By Name(w628) -> ("输入扭矩"=w627:sgl)
                        n492 = call "占空比.vi"() -> ("T1+T2"=w623:dbl, "T2"=w624:dbl, "T1"=w625:dbl)  [unwired: 9 in]
                        n493 = call-poly <userlib>:"MGI Running Average.vi"("Averaging Size"=w613, "Initialize? (F)"=w614, "Value"=w627) -> ("Average"=w618:sgl)  [unwired: 8 in]
                        n494 = call-poly <userlib>:"MGI Running Average.vi"("Averaging Size"=w613, "Initialize? (F)"=w614, "Value"=w623) -> ("Average"=w617:dbl)  [unwired: 8 in]
                        n495 = call-poly <userlib>:"MGI Running Average.vi"("Averaging Size"=w613, "Initialize? (F)"=w614, "Value"=w625) -> ("Average"=w615:dbl)  [unwired: 8 in]
                        n496 = call-poly <userlib>:"MGI Running Average.vi"("Averaging Size"=w613, "Initialize? (F)"=w614, "Value"=w624) -> ("Average"=w616:dbl)  [unwired: 8 in]
                        n497 = call "曲线采集.vi"("曲线引用"=w626, "曲线索引"=8, "X"=w618, "Y"=w617) -> ()  [unwired: 10 in, 2 out]
                        n498 = call "曲线采集.vi"("曲线引用"=w626, "曲线索引"=6, "X"=w618, "Y"=w615) -> ()  [unwired: 10 in, 2 out]
                        n499 = call "曲线采集.vi"("曲线引用"=w626, "曲线索引"=7, "X"=w618, "Y"=w616) -> ()  [unwired: 10 in, 2 out]
                      }
                    }
                    n500 = local write "力特性逆向去程"(w586) -> ()
                    n501 = local write "吸收电流"(w589) -> ()
                    n502 = local write "输入扭矩"(w587) -> ()
                    n503 = local write "输出扭矩(大)"(w588) -> ()
                    n504 = local write "T1+T2"(w590) -> ()
                    n505 = local write "T1"(w592) -> ()
                    n506 = local write "T2"(w591) -> ()
                  }
                  frame Enabled {
                  }
                }
              }
              frame 137 {
                n507 = disable-structure shown="禁用" {
                  frame Disabled {
                    n508 = global read "A180648.vi" "当前检测项"() -> (w632:T3)
                    n509 = case shown="\"手柄推拉力\"" w632 {
                      frame Default {
                      }
                      frame "手柄推拉力" {
                        n510 = call-poly "模式选择.vi"("Max Torque"=200.0, "Velocity"=sgl 1.0) -> ()  [unwired: 9 in, 1 out]
                      }
                    }
                  }
                  frame Enabled {
                  }
                }
                n511 = call "设备状态.vi"("枚举"=enum16{"Read", "Write"}."Write", "Status_Write"=i16 138 ("设备状态")) -> ()  [unwired: 9 in, 1 out]
                n512 = local write "STEP"("等待" ("STEP")) -> ()
              }
              frame 138 {
                n513 = disable-structure shown="禁用" {
                  frame Disabled {
                    n514 = control-ref of="管柱保持力试验"() -> (w640:refnum<vi>)
                    n515 = local read "当前车速"() -> (w637:i32)
                    n516 = global read "Global.vi" "传感器读数"() -> (w636:T9)
                    n517 = control-ref of="管柱推拉力试验"() -> (w638:refnum<vi>)
                    n518 = control-ref of="锁紧/开启"() -> (w639:refnum<vi>)
                    n519 = local read "力特性逆向回程"() -> (w641:bool)
                    n520 = case shown="100" w637 {
                      selector: w637 -> [w662 _]
                      tunnel: w636 -> [w667 w683]
                      tunnel: w638 -> [w666 _]
                      tunnel: w639 -> [_ w681]
                      tunnel: w640 -> [w664 _]
                      tunnel: w641 -> [w653 w669]
                      tunnel: [FALSE FALSE] -> w642
                      tunnel: [w654 w673] -> w643
                      tunnel: [w656 _] -> w644
                      tunnel: [w655 _] -> w645
                      tunnel: [_ w672] -> w646
                      tunnel: [_ w671] -> w647
                      tunnel: [_ w670] -> w648
                      tunnel: 10 -> [w652 w668]
                      frame 0, Default {
                        n521 = Unbundle By Name(w667) -> ("输入扭矩"=w665:sgl, "输出扭矩(大)"=w651:sgl, "吸收电流"=w663:sgl)
                        n522 = Multiply(x=w662, y=4) -> (x*y=w659:i32)
                        n523 = Subtract(x=w651, y=sgl 0.0) -> (x-y=w649:sgl)
                        n524 = call-poly <userlib>:"MGI Running Average.vi"("Averaging Size"=w652, "Initialize? (F)"=w653, "Value"=w663) -> ("Average"=w655:sgl)  [unwired: 8 in]
                        n525 = call-poly <userlib>:"MGI Running Average.vi"("Averaging Size"=w652, "Initialize? (F)"=w653, "Value"=w649) -> ("Average"=w656:sgl)  [unwired: 8 in]
                        n526 = call-poly <userlib>:"MGI Running Average.vi"("Averaging Size"=w652, "Initialize? (F)"=w653, "Value"=w665) -> ("Average"=w654:sgl)  [unwired: 8 in]
                        n527 = Add(x=w659, y=3) -> (x+y=w658:i32)
                        n528 = call "曲线采集.vi"("曲线引用"=w664, "曲线索引"=w658, "X"=w654, "Y"=w655) -> ()  [unwired: 10 in, 2 out]
                        n529 = call "曲线采集.vi"("曲线引用"=w666, "曲线索引"=w658, "X"=w654, "Y"=w656) -> ()  [unwired: 10 in, 2 out]
                      }
                      frame 100 {
                        n530 = Unbundle By Name(w683) -> ("输入扭矩"=w682:sgl)
                        n531 = call "占空比.vi"() -> ("T1+T2"=w678:dbl, "T2"=w679:dbl, "T1"=w680:dbl)  [unwired: 9 in]
                        n532 = call-poly <userlib>:"MGI Running Average.vi"("Averaging Size"=w668, "Initialize? (F)"=w669, "Value"=w682) -> ("Average"=w673:sgl)  [unwired: 8 in]
                        n533 = call-poly <userlib>:"MGI Running Average.vi"("Averaging Size"=w668, "Initialize? (F)"=w669, "Value"=w678) -> ("Average"=w672:dbl)  [unwired: 8 in]
                        n534 = call-poly <userlib>:"MGI Running Average.vi"("Averaging Size"=w668, "Initialize? (F)"=w669, "Value"=w680) -> ("Average"=w670:dbl)  [unwired: 8 in]
                        n535 = call-poly <userlib>:"MGI Running Average.vi"("Averaging Size"=w668, "Initialize? (F)"=w669, "Value"=w679) -> ("Average"=w671:dbl)  [unwired: 8 in]
                        n536 = call "曲线采集.vi"("曲线引用"=w681, "曲线索引"=11, "X"=w673, "Y"=w672) -> ()  [unwired: 10 in, 2 out]
                        n537 = call "曲线采集.vi"("曲线引用"=w681, "曲线索引"=9, "X"=w673, "Y"=w670) -> ()  [unwired: 10 in, 2 out]
                        n538 = call "曲线采集.vi"("曲线引用"=w681, "曲线索引"=10, "X"=w673, "Y"=w671) -> ()  [unwired: 10 in, 2 out]
                      }
                    }
                    n539 = local write "力特性逆向回程"(w642) -> ()
                    n540 = local write "吸收电流"(w645) -> ()
                    n541 = local write "输入扭矩"(w643) -> ()
                    n542 = local write "输出扭矩(大)"(w644) -> ()
                    n543 = local write "T1+T2"(w646) -> ()
                    n544 = local write "T1"(w648) -> ()
                    n545 = local write "T2"(w647) -> ()
                  }
                  frame Enabled {
                  }
                }
              }
              frame 139 {
                n546 = local read "布尔"() -> (w684:bool)
                n547 = case shown="真" w684 {
                  frame False {
                  }
                  frame True {
                    n548 = global read "A180648.vi" "车速"() -> (w688:sgl[])
                    n549 = local write "布尔"(FALSE ("布尔")) -> ()
                    n550 = Array Size(array=w688) -> (size(s)=w690:i32)
                    n551 = local read "当前车速"() -> (w687:i32)
                    n552 = Decrement(x=w690) -> (x-1=w686:i32)
                    n553 = Greater Or Equal?(x=w687, y=w686) -> (x >= y?=w689:bool)
                    n554 = case shown="真" w689 {
                      frame False {
                        n555 = stacked-sequence {
                          frame #0 {
                            n556 = local read "当前车速"() -> (w692:i32)
                            n557 = Increment(x=w692) -> (x+1=w691:i32)
                            n558 = local write "当前车速"(w691) -> ()
                          }
                          frame #1 {
                            w700 = u16 2 items=["byte", "word", "Dword"] ("数据类型")
                            w703 = u8 132 items=["I/O (P)"=128, "Input (I)"=129, "Output (Q)"=130, "Bit Memory (M)"=131, "Data (DB)"=132, "Instance Data (DI)"=133, "Local Data (L)"=134, "Predecessor Local Data (VL)"=135] ("寄存器类型")
                            n559 = local read "当前车速"() -> (w696:i32)
                            n560 = global read "A180648.vi" "车速"() -> (w697:sgl[])
                            n561 = Index Array(array=w697, index=w696) -> (element=w693:sgl)
                            n562 = Type Cast(type=u32 0, x=w693) -> (*(type *) &x=w698:u32)
                            n563 = Round Toward +Infinity(x=w693) -> (ceil(x): smallest int >= x=w695:sgl)
                            n564 = call "Write_Data.vi"("DB #"=u16 7, "寄存器类型"=w703, "写入数据"=w698, "数据类型"=w700, "写入地址"=u32 160) -> ()  [unwired: 4 in, 3 out]
                            n565 = To Unsigned Word Integer(number=w695) -> (unsigned 16bit integer=w694:u16)
                            n566 = global write "A180648.vi" "当前车速"(w694) -> ()
                          }
                          frame #2 {
                            n567 = call "设备状态.vi"("枚举"=enum16{"Read", "Write"}."Write", "Status_Write"=i16 132 ("设备状态")) -> ()  [unwired: 9 in, 1 out]
                          }
                          frame #3 {
                            n568 = disable-structure shown="禁用" {
                              frame Disabled {
                                n569 = global read "A180648.vi" "当前检测项"() -> (w706:T3)
                                n570 = case shown="\"手柄推拉力\"" w706 {
                                frame Default {
                                }
                                frame "手柄推拉力" {
                                n571 = call-poly "模式选择.vi"("Max Torque"=200.0, "Velocity"=sgl -1.0) -> ()  [unwired: 9 in, 1 out]
                                }
                                }
                              }
                              frame Enabled {
                              }
                            }
                          }
                          frame #4 {
                            w709 = TRUE
                            n572 = local write "力特性逆向回程"(w709) -> ()
                            n573 = local write "力特性正向去程"(w709) -> ()
                            n574 = local write "力特性逆向去程"(w709) -> ()
                            n575 = local write "力特性正向回程"(w709) -> ()
                          }
                        }
                      }
                      frame True {
                        n576 = local write "STEP"("判定" ("STEP")) -> ()
                      }
                    }
                  }
                }
              }
              frame 142 {
                n577 = stacked-sequence {
                  frame #0 {
                    n578 = global read "Global.vi" "输出占空比"() -> (w714:refnum<vi>)
                    n579 = call "设备状态.vi"("枚举"=enum16{"Read", "Write"}."Write", "Status_Write"=i16 143) -> ()  [unwired: 9 in, 1 out]
                    n580 = property class="Num"(reference=w714, "Val(Sgnl)"=52.0) -> ()  [unwired: 1 in, 2 out]
                  }
                  frame #1 {
                    n581 = Wait (ms)(milliseconds to wait=u32 2000 ("等待时间（毫秒）")) -> ()  [unwired: 1 out]
                  }
                }
              }
              frame 143 {
                n582 = disable-structure shown="禁用" {
                  frame Disabled {
                    n583 = stacked-sequence {
                      frame #0 {
                        n584 = control-ref of="振动1NVH-FFT"() -> (w720:refnum<vi>)
                        n585 = control-ref of="振动2NHV-FFT"() -> (w719:refnum<vi>)
                        n586 = call "振动检测.vi"("振动一"=w720, "通道输入"=tag "cDaq1Mod1/ai1:2" ("DAQmx物理通道"), "振动二"=w719, "重置"=FALSE) -> ("spectrum info"=w718:T10[])  [unwired: 10 in, 1 out]
                        n587 = global write "Global.vi" "spectrum info"(w718) -> ()
                      }
                      frame #1 {
                        n588 = global read "Global.vi" "输出占空比"() -> (w724:refnum<vi>)
                        n589 = call "设备状态.vi"("枚举"=enum16{"Read", "Write"}."Write", "Status_Write"=i16 144) -> ()  [unwired: 9 in, 1 out]
                        n590 = property class="Num"(reference=w724, "Val(Sgnl)"=48.0) -> ()  [unwired: 1 in, 2 out]
                      }
                      frame #2 {
                        n591 = Wait (ms)(milliseconds to wait=u32 2000 ("等待时间（毫秒）")) -> ()  [unwired: 1 out]
                      }
                    }
                  }
                  frame Enabled {
                  }
                }
              }
              frame 144 {
                n592 = disable-structure shown="禁用" {
                  frame Disabled {
                    n593 = stacked-sequence {
                      frame #0 {
                        n594 = control-ref of="振动1NVH-FFT"() -> (w730:refnum<vi>)
                        n595 = control-ref of="振动2NHV-FFT"() -> (w729:refnum<vi>)
                        n596 = call "振动检测.vi"("振动一"=w730, "通道输入"=tag "cDaq1Mod1/ai1:2" ("DAQmx物理通道"), "振动二"=w729, "重置"=FALSE) -> ("spectrum info"=w728:T10[])  [unwired: 10 in, 1 out]
                        n597 = global write "Global.vi" "spectrum info"(w728) -> ()
                      }
                      frame #1 {
                        n598 = call "设备状态.vi"("枚举"=enum16{"Read", "Write"}."Write", "Status_Write"=i16 145) -> ()  [unwired: 9 in, 1 out]
                      }
                    }
                  }
                  frame Enabled {
                  }
                }
              }
              frame 152 {
                n599 = global read "A180648.vi" "逆向空载试验参数"() -> (w735:T16)
                n600 = Unbundle By Name(w735) -> ("启用助力"=w734:dbl)  [unwired: 1 out]
                n601 = case shown="1" w734 {
                  frame 0, Default {
                    n602 = call "设备状态.vi"("枚举"=enum16{"Read", "Write"}."Write", "Status_Write"=i16 154 ("设备状态")) -> ()  [unwired: 9 in, 1 out]
                  }
                  frame 1 {
                    n603 = call "设备状态.vi"("枚举"=enum16{"Read", "Write"}."Write", "Status_Write"=i16 155 ("设备状态")) -> ()  [unwired: 9 in, 1 out]
                  }
                }
                n604 = local write "STEP"("等待" ("STEP")) -> ()
              }
              frame 154, 155 {
                n605 = disable-structure shown="禁用" {
                  frame Disabled {
                    n606 = global read "Global.vi" "逆向空载系数"() -> (w740:dbl)
                    n607 = call "传感器数据.vi"() -> ("电缸位移"=w755:sgl)  [unwired: 6 in, 5 out]
                    n608 = Unbundle By Name(w755) -> ("输出扭矩(大)"=w741)
                    n609 = local read "逆向空载正向初始化"() -> (w746:bool)
                    n610 = global read "A180648.vi" "逆向空载试验参数"() -> (w754:T16)
                    n611 = Multiply(x=w741, y=w740) -> (x*y=w742:dbl)
                    n612 = Subtract(x=w742, y=sgl 0.0) -> (x-y=w743:sgl)
                    n613 = Unbundle By Name(w754) -> ("试验速度"=w748:dbl, "试验角度"=w753:dbl, "保护扭矩"=w752:dbl, "启用助力"=w749:dbl)
                    n614 = call-poly <userlib>:"MGI Running Average.vi"("Averaging Size"=10, "Initialize? (F)"=w746, "Value"=w743) -> ("Average"=w747:sgl)  [unwired: 8 in]
                    n615 = Less Or Equal?(y=w753) -> (x <= y?=w751:bool)  [unwired: 1 in]
                    n616 = Less Or Equal?(x=w747, y=w752) -> (x <= y?=w750:bool)
                    n617 = And(x=w751, y=w750) -> ()  [unwired: 1 out]
                    n618 = case shown="假" {
                      selector: _ -> [_ _]
                      tunnel: w747 -> [_ w767]
                      tunnel: w749 -> [w757 _]
                      tunnel: w748 -> [w756 _]
                      frame False {
                        n619 = stacked-sequence {
                          tunnel: w757 -> [_ w758 _ _]
                          tunnel: w756 -> [_ _ w763 _]
                          frame #0 {
                          }
                          frame #1 {
                            n620 = case shown="0, 默认" w758 {
                              frame 0, Default {
                                n621 = call "设备状态.vi"("枚举"=enum16{"Read", "Write"}."Write", "Status_Write"=i16 156 ("设备状态")) -> ()  [unwired: 9 in, 1 out]
                              }
                              frame 1 {
                                n622 = call "设备状态.vi"("枚举"=enum16{"Read", "Write"}."Write", "Status_Write"=i16 157 ("设备状态")) -> ()  [unwired: 9 in, 1 out]
                              }
                            }
                          }
                          frame #2 {
                            (unwired) FALSE ("Reset Count")
                            (unwired) 50.0 ("Max Torque")
                            n623 = Negate(x=w763) -> ()  [unwired: 1 out]
                          }
                          frame #3 {
                            n624 = local write "STEP"("等待" ("STEP")) -> ()
                          }
                        }
                      }
                      frame True {
                        n625 = control-ref of="逆向空载试验"() -> (w769:refnum<vi>)
                        n626 = call "曲线采集.vi"("曲线引用"=w769, "曲线索引"=0, "Y"=w767) -> ("错误输出"=w766:errorcluster)  [unwired: 11 in, 1 out]
                        n627 = Unbundle By Name(w766) -> ("status"=w765:bool)
                        n628 = local write "逆向空载正向初始化"(w765) -> ()
                      }
                    }
                  }
                  frame Enabled {
                  }
                }
              }
              frame 156, 157 {
                n629 = disable-structure shown="禁用" {
                  frame Disabled {
                    w776 = 10 ("Averaging Size")
                    n630 = global read "A180648.vi" "逆向空载试验参数"() -> (w784:T16)
                    n631 = call "传感器数据.vi"() -> ("电缸位移"=w774:sgl)  [unwired: 6 in, 5 out]
                    n632 = global read "Global.vi" "逆向空载系数"() -> (w772:dbl)
                    n633 = Unbundle By Name(w774) -> ("输出扭矩(大)"=w773)
                    n634 = local read "锁紧/开启初始化"() -> (w777:bool)
                    n635 = Unbundle By Name(w784) -> ("保护扭矩"=w783:dbl)
                    n636 = Multiply(x=w773, y=w772) -> (x*y=w771:dbl)
                    n637 = Subtract(x=w771, y=sgl 0.0) -> (x-y=w770:sgl)
                    n638 = Negate(x=w783) -> (-x=w780:dbl)
                    n639 = call-poly <userlib>:"MGI Running Average.vi"("Averaging Size"=w776, "Initialize? (F)"=w777) -> ("Average[i]"=w778:dbl[])  [unwired: 9 in]
                    n640 = call-poly <userlib>:"MGI Running Average.vi"("Averaging Size"=w776, "Initialize? (F)"=w777, "Value"=w770) -> ("Average"=w779:sgl)  [unwired: 8 in]
                    n641 = Greater Or Equal To 0?(x=w778) -> (x >= 0?=w782:bool[])
                    n642 = Greater Or Equal?(x=w779, y=w780) -> (x >= y?=w781:bool)
                    n643 = And(x=w782, y=w781) -> ()  [unwired: 1 out]
                    n644 = case shown="假" {
                      selector: _ -> [_ _]
                      tunnel: w778 -> [_ _]
                      tunnel: w779 -> [_ w788]
                      frame False {
                        n645 = stacked-sequence {
                          frame #0 {
                          }
                          frame #1 {
                            n646 = local write "STEP"("判定" ("STEP")) -> ()
                          }
                        }
                      }
                      frame True {
                        n647 = control-ref of="逆向空载试验"() -> (w790:refnum<vi>)
                        n648 = call "曲线采集.vi"("曲线引用"=w790, "曲线索引"=1, "Y"=w788) -> ("错误输出"=w787:errorcluster)  [unwired: 11 in, 1 out]
                        n649 = Unbundle By Name(w787) -> ("status"=w786:bool)
                        n650 = local write "锁紧/开启初始化"(w786) -> ()
                      }
                    }
                  }
                  frame Enabled {
                  }
                }
              }
              frame 999 {
                n651 = call "浮动通知.vi"("通知内容"="请启动！" ("Status")) -> ()  [unwired: 11 in]
              }
              frame 1000 {
                n652 = local write "STEP"("初始化" ("STEP")) -> ()
              }
              frame 1024 {
                n653 = call "停止发送CAN.vi"() -> ()  [unwired: 11 in, 1 out]
                n654 = local write "STEP"("退出自动" ("STEP")) -> ()
              }
              frame Default {
              }
            }
          }
          frame "合格判定" {
            n655 = Wait (ms)(milliseconds to wait=u32 100 ("等待时间（毫秒）")) -> ()  [unwired: 1 out]
            n656 = local write "STEP"("等待" ("STEP")) -> ()
          }
          frame "报表" {
            n657 = stacked-sequence {
              seq-local: [_ w797 _ _] -> [_ _ w802 _]
              frame #0 {
                n658 = global write "Global.vi" "计时开始"(FALSE ("计时开始")) -> ()
              }
              frame #1 {
                n659 = global read "Global.vi" "产品编号"() -> (w798:string)
                n660 = call "Report.vi"("文件重命名"=TRUE, "文件名称"=w798, "检测结果"="判定结果") -> ("PRODUCT_VAULE"=w797:string)  [unwired: 7 in, 1 out]
              }
              frame #2 {
                n661 = global read "Global.vi" "联机模式"() -> (w801:enum16{"单机", "追溯"})
                n662 = case shown="\"追溯\"" w801 {
                  tunnel: w802 -> [_ w803]
                  frame "单机", Default {
                  }
                  frame "追溯" {
                    n663 = global read "Global.vi" "Result"() -> (w805:refnum<vi>)
                    n664 = property class="Tbl"(reference=w805) -> (reference out=w810:refnum<vi>, error out=w807:errorcluster, "Row Headers[]"=w808:string[])  [unwired: 1 in]
                    n665 = property class="Tbl"(reference=w810, error in=w807) -> (error out=w806:errorcluster, "Value"=w809:string[][])  [unwired: 1 out]
                    n666 = for {
                      tunnel: w809 -> [w817] mode=indexing
                      tunnel: w808 -> [w818] mode=indexing
                      tunnel: [w815] -> w804 mode=indexing if=w816
                      shift-right: [w814] -> _
                      shift-left: w806 -> [w814]
                      n667 = Build Array (concatenate)(w818, w817) -> (w815:string[])
                      n668 = Index Array(array=w817) -> (element=w819:string)  [unwired: 1 in]
                      n669 = case shown="\"\"" w819 {
                        tunnel: [TRUE FALSE] -> w816
                        frame Default {
                        }
                        frame "" {
                        }
                      }
                    }
                    n670 = global read "追溯Global.vi" "DEVICE_ID"() -> (w812:string)
                    n671 = global read "追溯Global.vi" "CODE_ID"() -> (w813:string)
                    n672 = global read "追溯Global.vi" "USER_ID"() -> (w811:string)
                    n673 = call "UPTEST.vi"("Result"=w804, "CODE_ID"=w813, "DEVICE_ID"=w812) -> ()  [unwired: 6 in, 1 out]
                    n674 = call "UPRESULT.vi"("DEVICE_ID"=w812, "USER_ID"=w811, "CODE_ID"=w813, "RESULT_VALUE"=w803) -> ()  [unwired: 11 in, 1 out]
                  }
                }
              }
              frame #3 {
                n675 = local write "STEP"("进入自动" ("STEP")) -> ()
              }
            }
          }
        }
        n676 = global read "Global.vi" "程序关闭"() -> (w24:bool)
      }
      n677 = while {
        shift-right: [w823] -> w22
        shift-left: w21 -> [w824]
        stop <- w825 stop-if-true
        n678 = event shown="[3] \"管柱保持力试验\", \"锁紧/开启\", \"管柱推拉力试验\", \"手柄锁紧力试验\", \"手柄开启力试验\", \"逆向空载试验\": 标尺范围更改" {
          selector: w824 -> [_ _ _ _ _ _ _]
          dyn-events: [_ _ _ _ _ _ _] -> w823
          timeout: 200 -> [_ _ _ _ _ _ _]
          event Timeout {
            n679 = event-data() -> ()  [unwired: 1 in, 3 out]
            n680 = call "Obtain Broadcast Events for Registration.vi"() -> ("Already running?"=w827:bool)  [unwired: 9 in, 2 out]
            n681 = case shown="真" w827 {
              frame False {
                n682 = local write "STEP"("手动" ("STEP")) -> ()
              }
              frame True {
                n683 = call "错误代码.vi"() -> ("Status_Read"=w829:u32)  [unwired: 11 in]
                n684 = feedback #1() -> (w839:u32)  [unwired: 1 in]
                n685 = feedback-in #1(w829) -> ()
                n686 = case shown="0" w829 {
                  frame 0 {
                    n687 = global read "Global.vi" "报警图标"() -> (w840:refnum<vi>)
                    n688 = property class="Bool"(reference=w840, "Visible"=FALSE ("可见")) -> ()  [unwired: 1 in, 2 out]
                  }
                  frame 1, Default {
                    n689 = global read "Global.vi" "报警图标"() -> (w843:refnum<vi>)
                    n690 = property class="Bool"(reference=w843, "Visible"=TRUE ("可见")) -> ()  [unwired: 1 in, 2 out]
                  }
                }
                n691 = Greater Or Equal?(x=w829, y=i16 5000) -> (x >= y?=w837:bool)
                n692 = Less?(x=w829, y=i16 5200) -> (x < y?=w838:bool)
                n693 = Equal?(x=w829, y=w839) -> (x = y?=w836:bool)
                n694 = global read "Global.vi" "报警图标"() -> (w831:refnum<vi>)
                n695 = And(x=w837, y=w838) -> (x .and. y?=w830:bool)
                n696 = property class="Bool"(reference=w831, "Value"=w830) -> ()  [unwired: 1 in, 2 out]
                n697 = Bundle By Name(cluster=errorcluster {"status"=FALSE, "code"=0, "source"=""} ("错误常量"), "status"=w830, "code"=w829) -> (w835:errorcluster)
                n698 = case shown="假" w836 {
                  tunnel: w835 -> [w844 _]
                  frame False {
                    n699 = call "报警处理.vi"("错误常量"=w844) -> ()  [unwired: 9 in, 2 out]
                  }
                  frame True {
                  }
                }
              }
            }
          }
          event User Event {
            n700 = event-data() -> ("试验项"=→"试验项目":T1)  [unwired: 1 in]
            n701 = disable-structure shown="禁用" {
              frame Disabled {
                n702 = local read "管柱保持力试验"() -> (w849:cluster{dbl[], dbl[]}[])
                n703 = global read "判定参数.vi" "最大位移"() -> (w846:dbl)
                n704 = global read "判定参数.vi" "最大拉力"() -> (w848:dbl)
                n705 = global read "判定参数.vi" "最小拉力"() -> (w847:dbl)
                n706 = for {
                  tunnel: [w856] -> w850 mode=indexing
                  tunnel: w849 -> [w855] mode=indexing
                  tunnel: w848 -> [w854]
                  tunnel: w847 -> [w853]
                  tunnel: w846 -> [w852]
                  tunnel: w846 -> [w851]
                  i -> [w857]
                  n707 = case shown="1" w857 {
                    tunnel: [w858 w859] -> w856
                    tunnel: w855 -> [w858 _]
                    tunnel: w854 -> [_ w863]
                    tunnel: w853 -> [_ w862]
                    tunnel: w852 -> [_ w861]
                    tunnel: w851 -> [_ w860]
                    frame 0, Default {
                    }
                    frame 1 {
                      n708 = Build Array(w861, w861, w860, w860, w861) -> (w865:dbl[])
                      n709 = Build Array(w862, w863, w863, w862, w862) -> (w864:dbl[])
                      n710 = Bundle(w865, w864) -> (w859:cluster{dbl[], dbl[]})  [unwired: 1 in]
                    }
                  }
                }
                n711 = local write "管柱保持力试验"(w850) -> ()
              }
              frame Enabled {
              }
            }
            n712 = disable-structure shown="禁用" {
              disable-tunnel: _ -> [w866 _]
              frame Disabled {
                n713 = global read "A180648.vi" "检测结果"() -> (w869:string[][][])
                n714 = global read "Global.vi" "Result"() -> (w867:refnum<vi>)
                n715 = Index Array(array=w869, index (dim 0)=w866) -> (element=w868:string[][])  [unwired: 2 in]
                n716 = property class="Tbl"(reference=w867, "Value"=w868) -> ()  [unwired: 1 in, 2 out]
              }
              frame Enabled {
              }
            }
          }
          event "试验项目": Value Change {
            n717 = event-data() -> ("NewVal"=w870:T1)  [unwired: 1 in]
            n718 = disable-structure shown="禁用" {
              disable-tunnel: w870 -> [w874 _]
              frame Disabled {
                n719 = global read "A180648.vi" "检测结果"() -> (w873:string[][][])
                n720 = global read "Global.vi" "Result"() -> (w871:refnum<vi>)
                n721 = Index Array(array=w873, index (dim 0)=w874) -> (element=w872:string[][])  [unwired: 2 in]
                n722 = property class="Tbl"(reference=w871, "Value"=w872) -> ()  [unwired: 1 in, 2 out]
              }
              frame Enabled {
              }
            }
          }
          event "管柱保持力试验", "锁紧/开启", "管柱推拉力试验", "手柄锁紧力试验", "手柄开启力试验", "逆向空载试验": Scale Range Change {
            n723 = event-data() -> ("CtlRef"=w875:refnum<vi>)  [unwired: 1 in, 4 out]
            n724 = disable-structure shown="禁用" {
              disable-tunnel: w875 -> [w876 _]
              frame Disabled {
                n725 = call "XY_conf.vi"("方式"=enum16{"写入", "读取"}."写入", "XY图引用"=w876) -> ()  [unwired: 3 in, 1 out]
              }
              frame Enabled {
              }
            }
          }
          event Panel Close {
            n726 = event-data() -> ()  [unwired: 1 in, 4 out]
            n727 = global write "Global.vi" "程序关闭"(TRUE ("程序关闭")) -> ()
          }
          event "管柱保持力试验", "锁紧/开启", "管柱推拉力试验", "振动1NVH-FFT", "手柄锁紧力试验", "手柄开启力试验", "逆向空载试验": Mouse Enter; "管柱保持力试验", "锁紧/开启", "管柱推拉力试验", "振动1NVH-FFT", "手柄锁紧力试验", "手柄开启力试验", "逆向空载试验": Mouse Leave; "管柱保持力试验", "锁紧/开启", "管柱推拉力试验", "振动1NVH-FFT", "手柄锁紧力试验", "手柄开启力试验", "逆向空载试验": Cursor Move {
            n728 = event-data() -> ("CtlRef"=w881:refnum<vi>, "Type"=w879:T17)  [unwired: 1 in]
            n729 = call "CursorShow.vi"("nameShow"=TRUE, "Type"=w879, "Graph"=w881) -> ()  [unwired: 7 in, 2 out]
          }
          event "管柱保持力试验", "锁紧/开启", "管柱推拉力试验", "振动1NVH-FFT", "手柄锁紧力试验", "手柄开启力试验", "逆向空载试验": Mouse Down {
            n730 = event-data() -> ("CtlRef"=w886:refnum<vi>, "Coords"=w885:T18, "Type"=w883:T17)  [unwired: 1 in]
            n731 = invoke class="WFGraph" method="Map Coords To XY"(reference=w886, "Coords"=w885) -> (reference out=w884:refnum<vi>, "XY"=w882:cluster{"X":dbl, "Y":dbl})  [unwired: 5 in, 5 out]
            n732 = call "CursorShow.vi"("游标.游标位置"=w882, "Type"=w883, "Graph"=w884) -> ()  [unwired: 7 in, 2 out]
          }
        }
        n733 = global read "Global.vi" "程序关闭"() -> (w825:bool)
      }
    }
  }
  n734 = Unregister For Events(event registration refnum=w4) -> ()  [unwired: 1 in, 1 out]
